vi "UNO_01.vi"() -> ()   [LabVIEW 2011]
uses:
  <vilib>/LabVIEW Interface for Arduino/Type Defs/Analog Pin.ctl
  <vilib>/LabVIEW Interface for Arduino/LabVIEW Interface for Arduino.lvlib
  <vilib>/Analysis/NI_AALBase.lvlib
panel:
  out "appended array 2":dbl[][](array[numeric])
  out "appended array":dbl[][](array[numeric])
  out "t":dbl[](array[numeric])
  out "path RLC":path
  out "MEASURE V [V]":dbl
  out "MEASURE I [A]":dbl
  out "MEASURE I [A]   2":dbl
  out "MEASURE V [V]  2":dbl
  out "MEASURE I [A]   8":dbl
  out "MEASURE V [V]  8":dbl
  out "MEASURE I [A]   7":dbl
  out "MEASURE V [V]  7":dbl
  out "MEASURE I [A]   6":dbl
  out "MEASURE V [V]  6":dbl
  out "MEASURE I [A]   5":dbl
  out "MEASURE V [V]  5":dbl
  out "MEASURE I [A]   4":dbl
  out "MEASURE V [V]  4":dbl
  out "MEASURE I [A]   3":dbl
  out "MEASURE V [V]  3":dbl
  out "MEASURE V [V]  16":dbl
  out "MEASURE I [A]   16":dbl
  out "MEASURE V [V]  15":dbl
  out "MEASURE I [A]   15":dbl
  out "MEASURE V [V]  14":dbl
  out "MEASURE I [A]   14":dbl
  out "MEASURE V [V]  13":dbl
  out "MEASURE I [A]   13":dbl
  out "MEASURE V [V]  12":dbl
  out "MEASURE I [A]   12":dbl
  out "MEASURE V [V]  11":dbl
  out "MEASURE I [A]   11":dbl
  out "MEASURE V [V]  10":dbl
  out "MEASURE I [A]   10":dbl
  out "MEASURE V [V]  9":dbl
  out "MEASURE I [A]   9":dbl
  out "RLC300 - digimess":string
  in  "dados":string
  in  "Tab Control":enum32{"Page 1", "Page 2"}(tab)
  out "Waveform Chart 2":dynamicdata(graph)
  out "Waveform Chart":dynamicdata(graph)
  in  "Analog Pin A":T1
  out "Voltage A":dbl(knob) scale=0.0..5.0
  in  "Analog Pin B":T1
  in  "Analog Pin C":T1
  out "Voltage B":dbl(knob) scale=0.0..5.0
  out "Voltage C":dbl(knob) scale=0.0..5.0
  out "Analog Port":dbl[](array[numeric])
  out "Resistencia":dbl
  out "Temperatura":dbl
  out "mean 2":dbl format="%.3p"
  in  "Refresh Button":bool
  out "Waveform Chart P 2":dbl[][](graph)
  out "C-50-N":bool
  out "C-50-L":bool
  out "Time":timestamp format="%<%X\n%x>T"
  out "Waveform Chart T":dynamicdata(graph)
  out "Waveform Chart P":dynamicdata(graph)
  out "Temperature (ºC)":dbl format="%#_4g"
  out "Pressure (bar)":dbl format="%#_4g"
  in  "New":bool
  in  "File name":string
  in  "Nota 01":string
  in  "Nota 2":string
  in  "Nota 3":string
  out "path":path
  in  "Sample name":string
  in  "Save Data":bool
  in  "Ajute P":dbl
  in  "Ajute T":dbl
  in  "Time (sec)":dbl
  in  "Stop":bool
  in  "New Button":bool
  in  "RLC":bool
  in  "Ligar RLC":bool
  in  "Close RLC 2":bool
  in  "read RLC":bool
  out "MEASURE A":dbl
  out "MEASURE B":dbl
  out "MEASURE B 2":dbl
  out "MEASURE A 2":dbl
  out "MEASURE B 8":dbl
  out "MEASURE A 8":dbl
  out "MEASURE B 7":dbl
  out "MEASURE A 7":dbl
  out "MEASURE B 6":dbl
  out "MEASURE A 6":dbl
  out "MEASURE B 5":dbl
  out "MEASURE A 5":dbl
  out "MEASURE B 4":dbl
  out "MEASURE A 4":dbl
  out "MEASURE B 3":dbl
  out "MEASURE A 3":dbl
  out "MEASURE B 9":dbl
  out "MEASURE A 9":dbl
  out "MEASURE B 10":dbl
  out "MEASURE A 10":dbl
  out "MEASURE B 11":dbl
  out "MEASURE A 11":dbl
  out "MEASURE B 12":dbl
  out "MEASURE A 12":dbl
  out "MEASURE B 13":dbl
  out "MEASURE A 13":dbl
  out "MEASURE B 14":dbl
  out "MEASURE A 14":dbl
  out "MEASURE B 15":dbl
  out "MEASURE A 15":dbl
  out "MEASURE B 16":dbl
  out "MEASURE A 16":dbl
  out "C-100-L":bool
  out "C-100-N":bool
  out "C-1K-L":bool
  out "C-1K-N":bool
  out "C-10K-L":bool
  out "C-10K-N":bool
  out "Z-50-L":bool
  out "Z-50-N":bool
  out "Z-100-L":bool
  out "Z-100-N":bool
  out "Z-1K-L":bool
  out "Z-1K-N":bool
  out "Z-10K-L":bool
  out "Z-10K-N":bool
  out "SET":dbl format="%#_3g"
  out "Waveform Chart P 3":dbl[][](graph)
  out "mean":dbl format="%.3p"
  out "mean 8":dbl format="%.3p"
  out "mean 7":dbl format="%.3p"
  out "mean 6":dbl format="%.3p"
  out "mean 5":dbl format="%.3p"
  out "mean 4":dbl format="%.3p"
  out "mean 3":dbl format="%.3p"
  out "mean 9":dbl format="%.3p"
  out "mean 10":dbl format="%.3p"
  out "mean 11":dbl format="%.3p"
  out "mean 12":dbl format="%.3p"
  out "mean 13":dbl format="%.3p"
  out "mean 14":dbl format="%.3p"
  out "mean 15":dbl format="%.3p"
  out "mean 16":dbl format="%.3p"
  # "C ( F )"
  # "R ( Ohm )"
  # "Z ( Ohm )"
  # "Phase ( deg)"
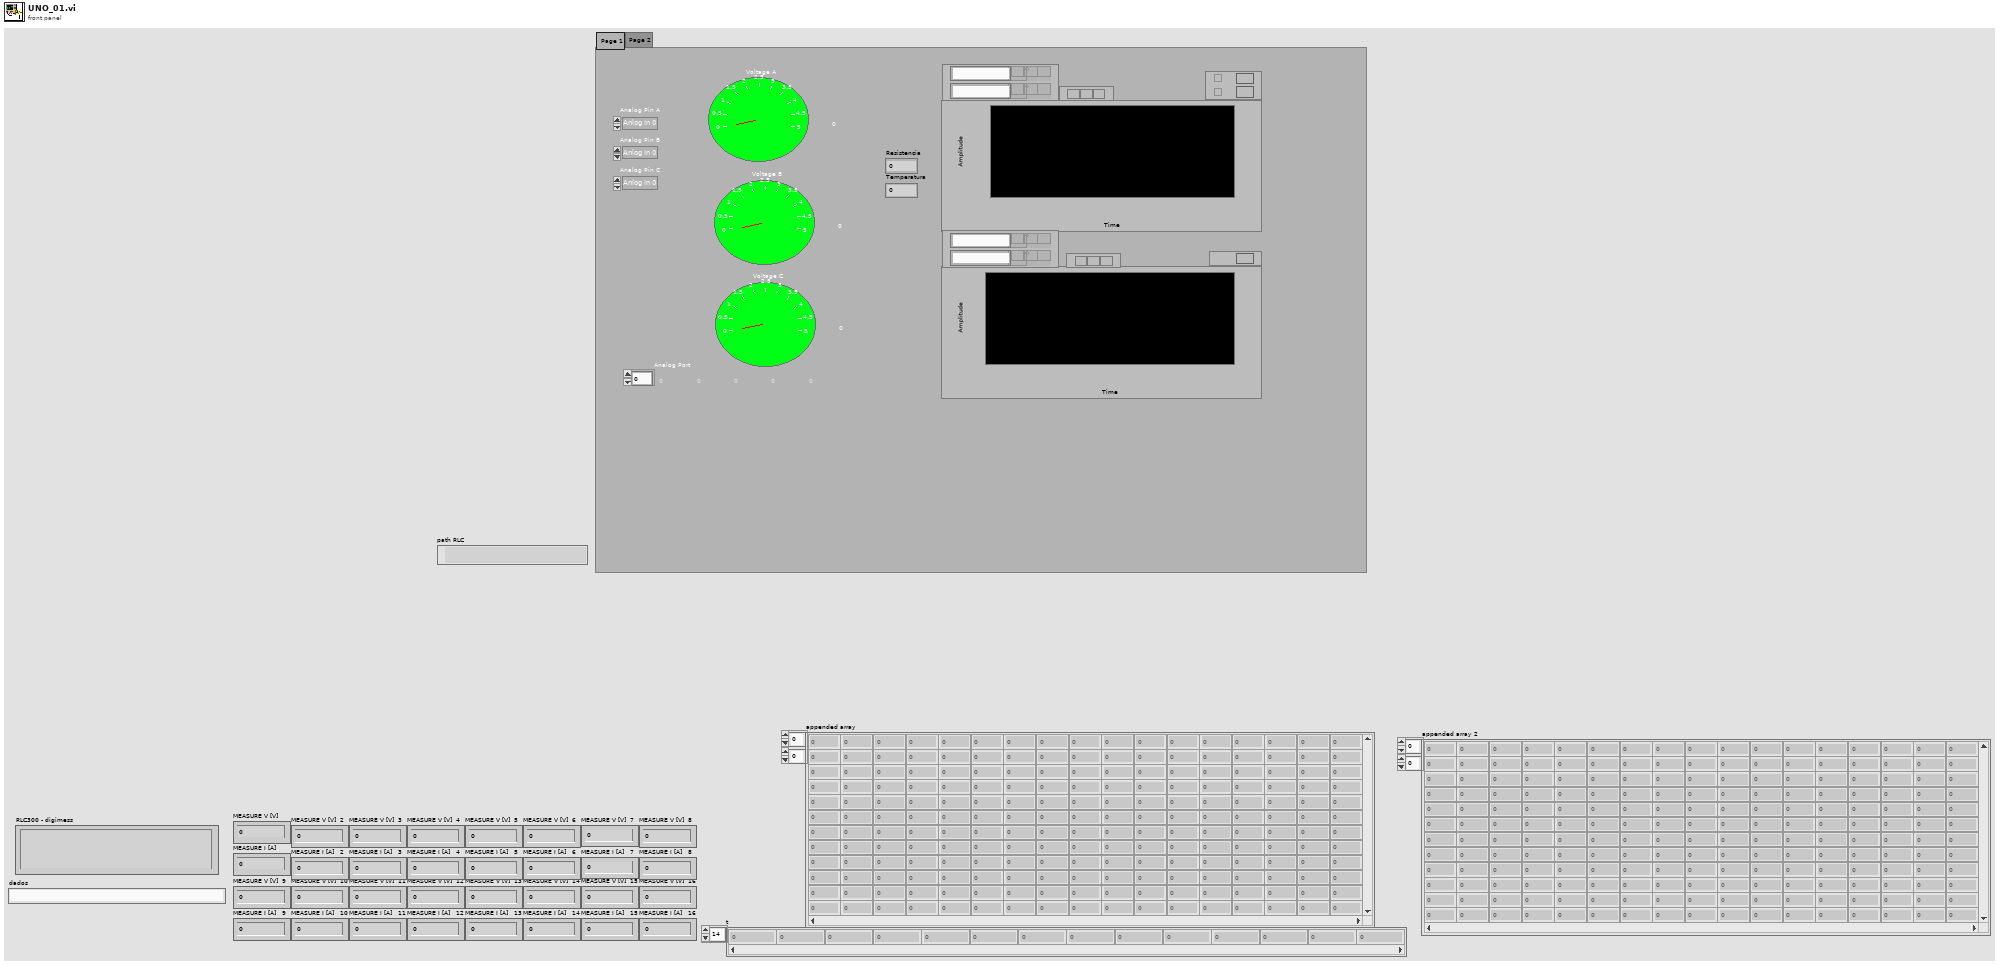
[diagram p1: front panel]
types:
  T1 = typedef "LabVIEW Interface for Arduino.lvlib/Analog Pin.ctl" = enum8{"Anlog In 0", "Anlog In 1", "Anlog In 2", "Anlog In 3", "Anlog In 4", "Anlog In 5"}
  T2 = typedef "LabVIEW Interface for Arduino.lvlib/Arduino Resource.ctl" = cluster{"VISA resource":refnum<visa-resource-name>, "Board Type":T3, "Connection Type":enum8{"USB / Serial"}, "Bytes Per Packet (15)":u8}
  T3 = typedef "LabVIEW Interface for Arduino.lvlib/Board Type.ctl" = enum16{"Uno", "Dimuelanove w/Atmega 328", "Mega 2560"}
  T4 = enum16{"open", "replace", "create", "open or create", "replace or create", "replace or create with confirmation"}
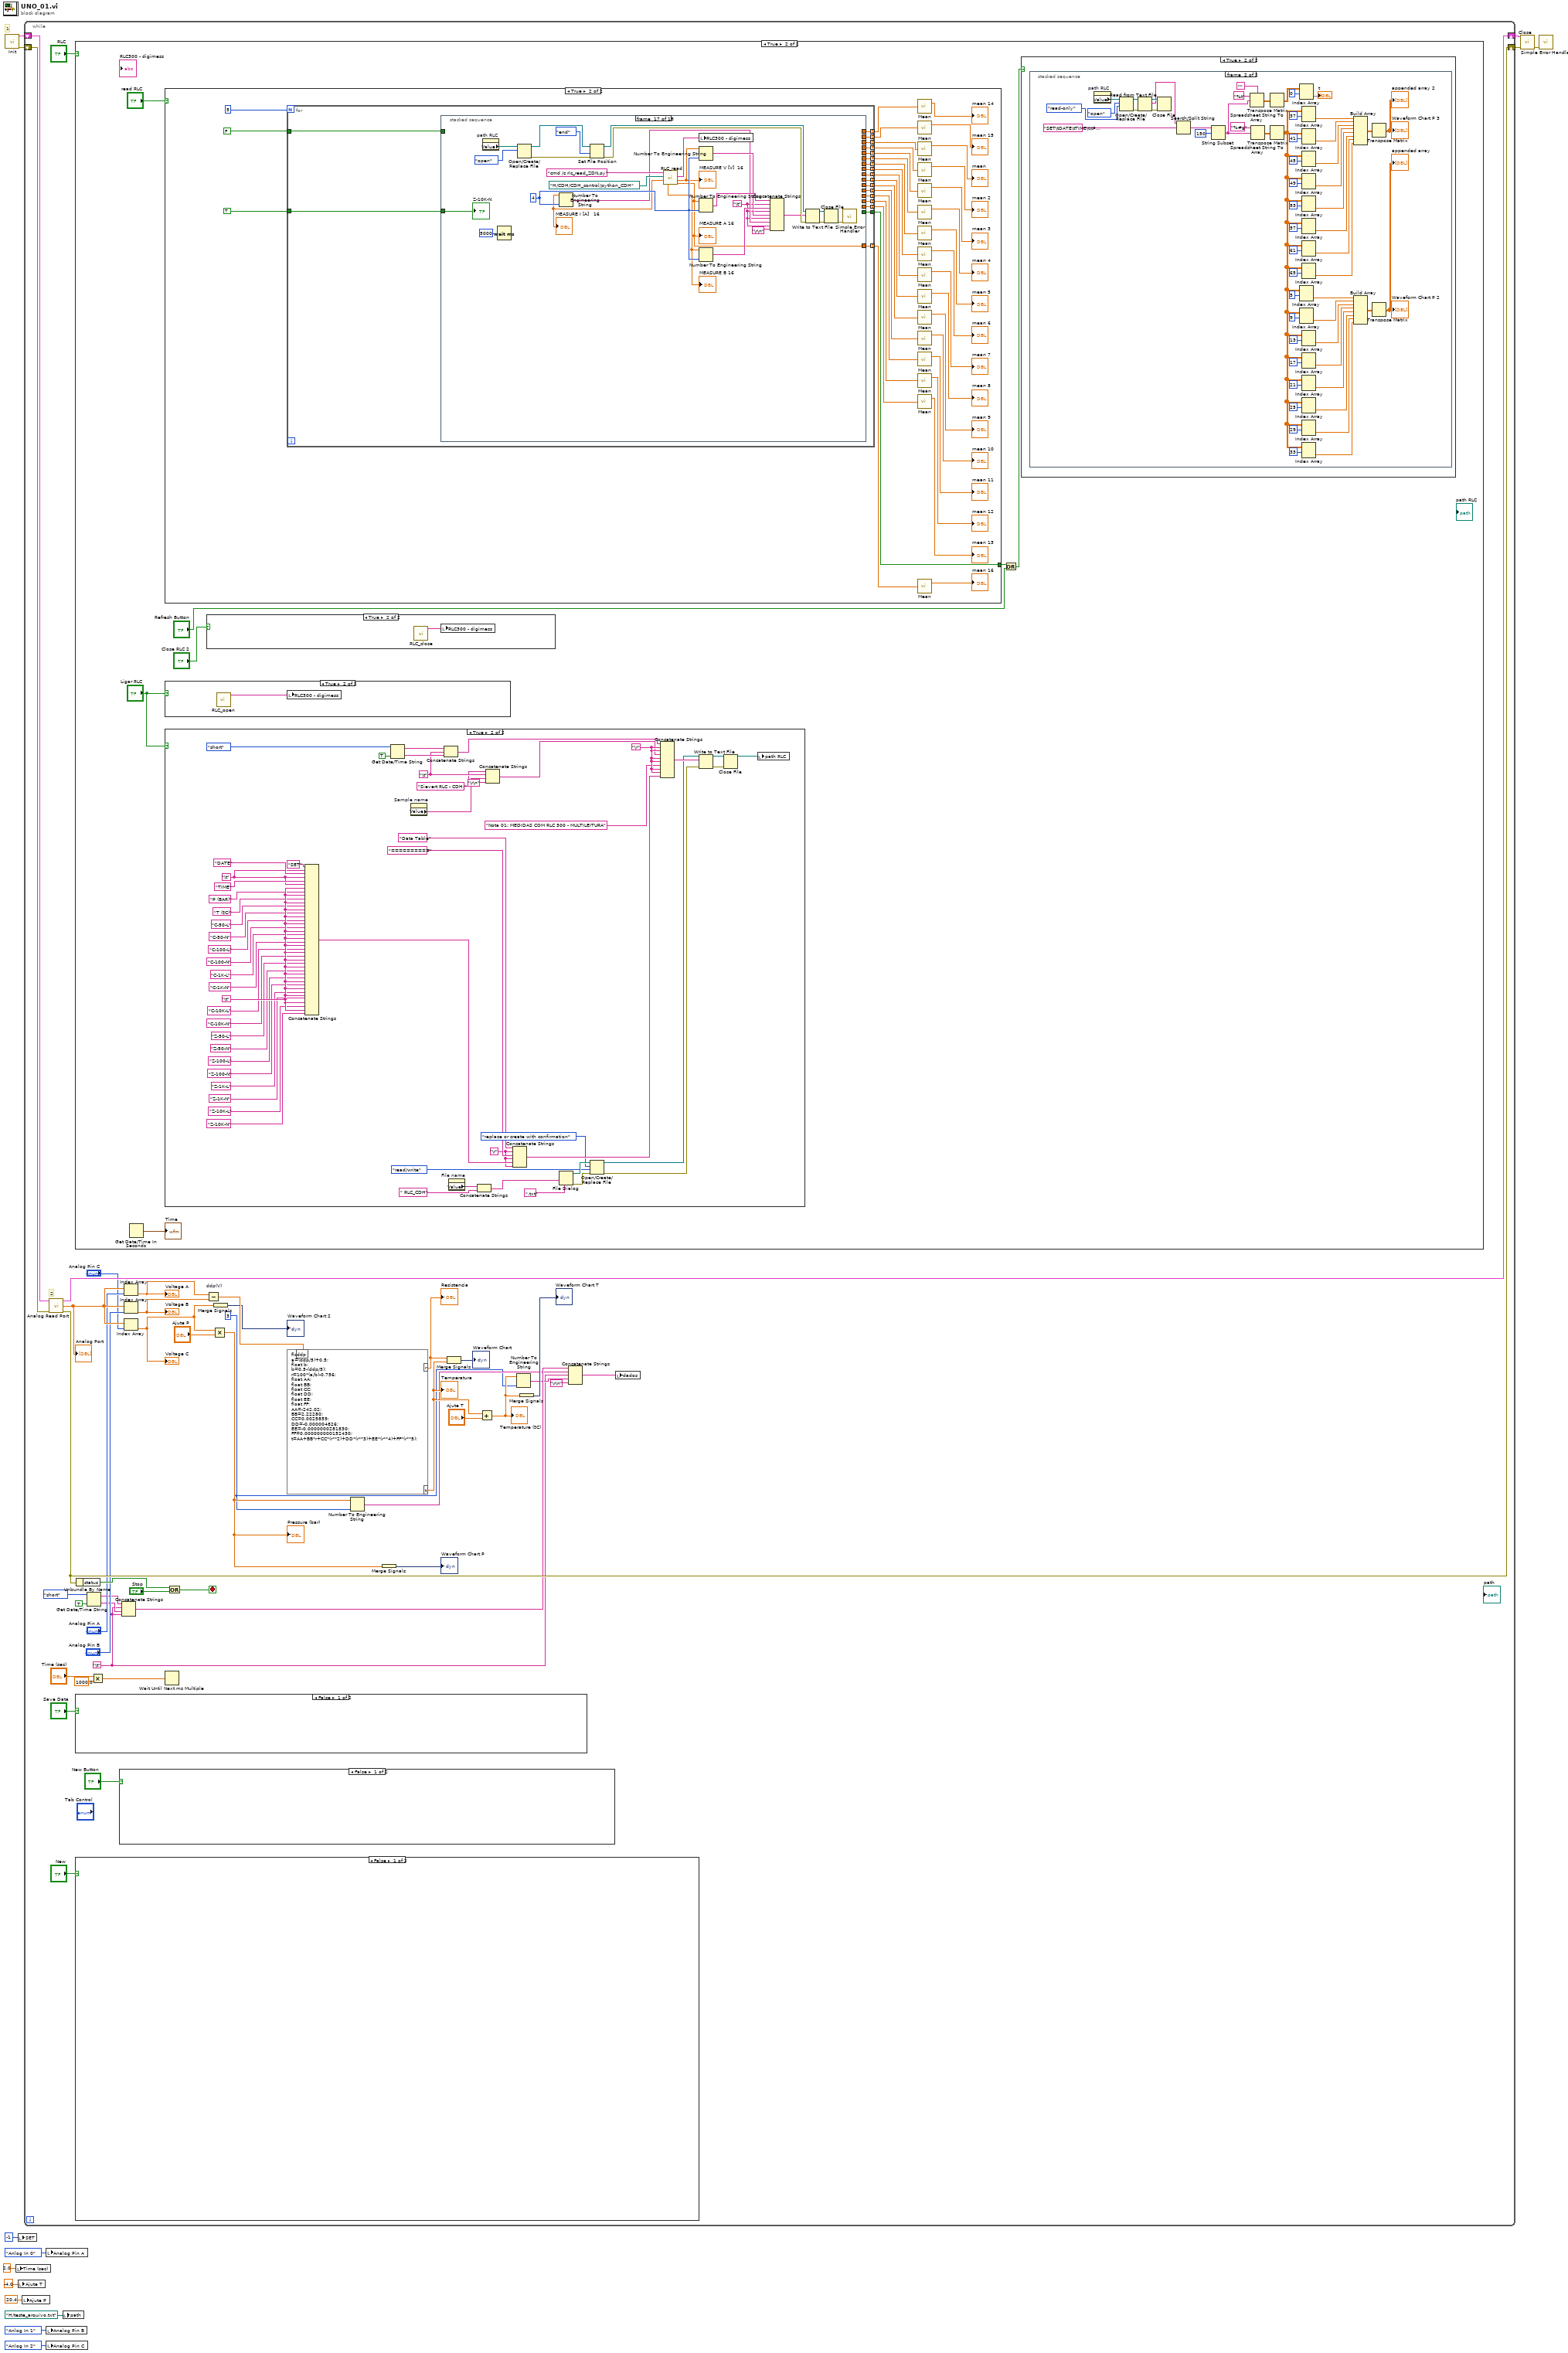
[diagram p0: block diagram]
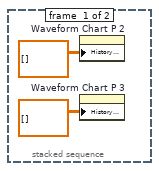
[diagram p4: hidden frame]
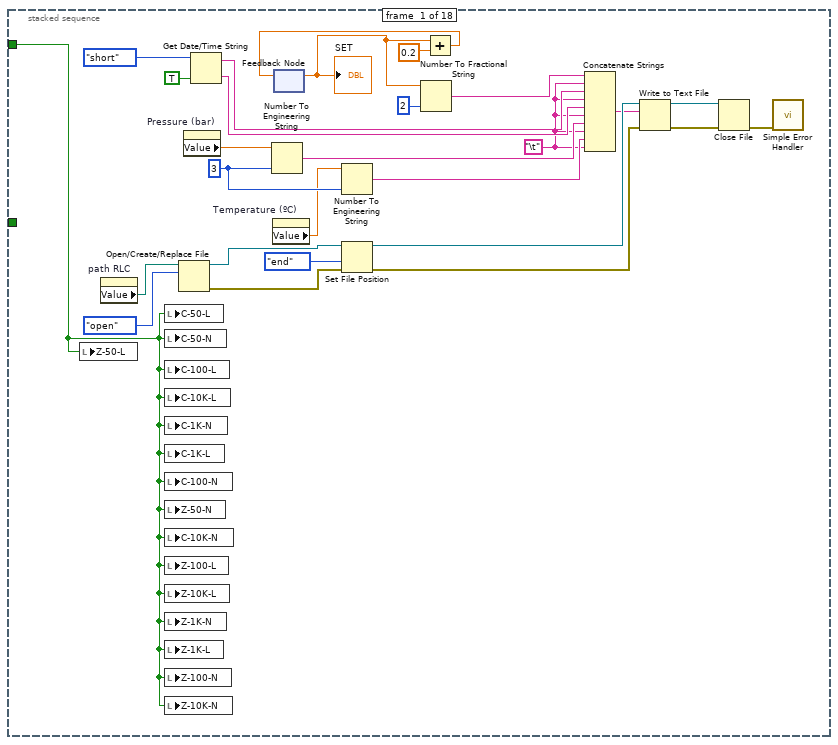
[diagram p7: hidden frame]
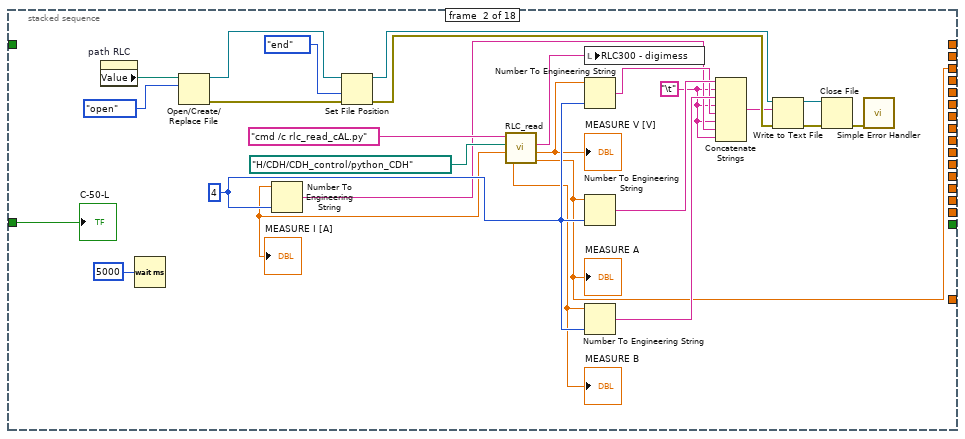
[diagram p8: hidden frame]
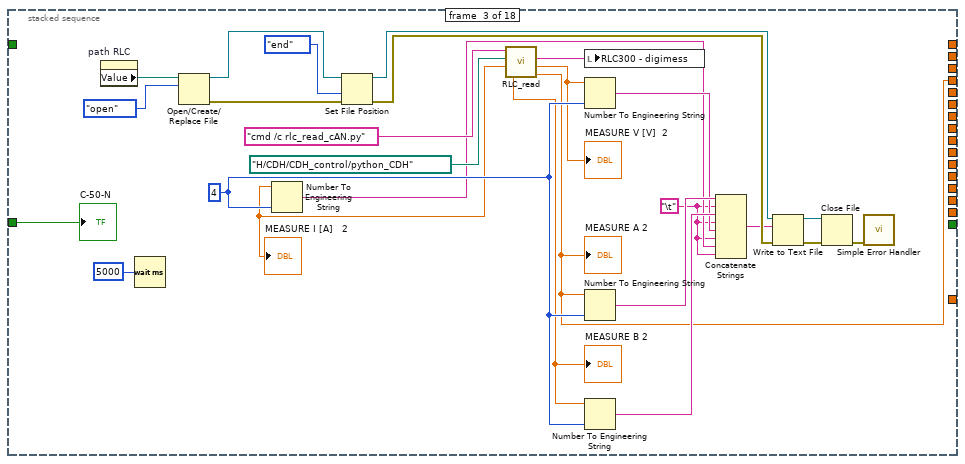
[diagram p9: hidden frame]
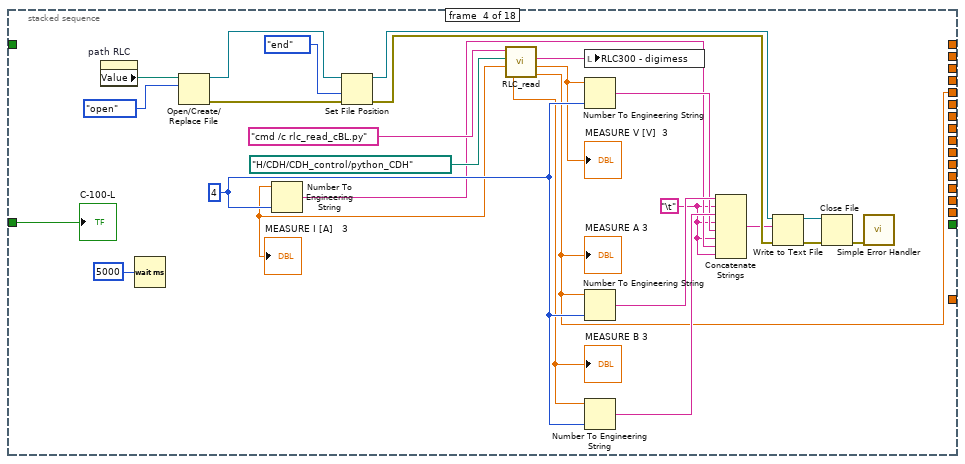
[diagram p10: hidden frame]
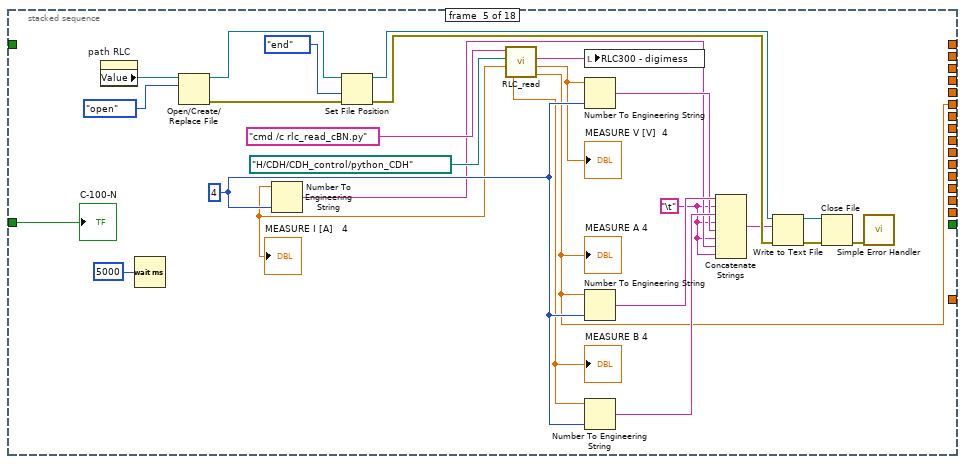
[diagram p11: hidden frame]
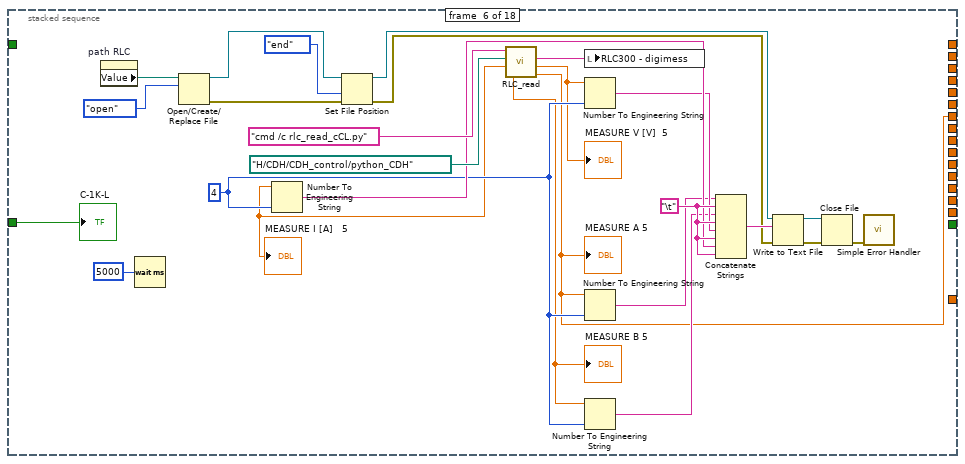
[diagram p12: hidden frame]
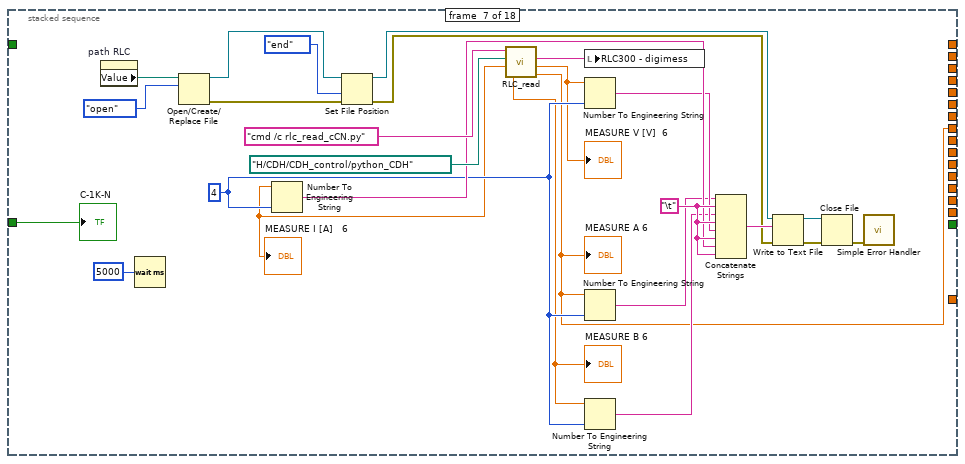
[diagram p13: hidden frame]
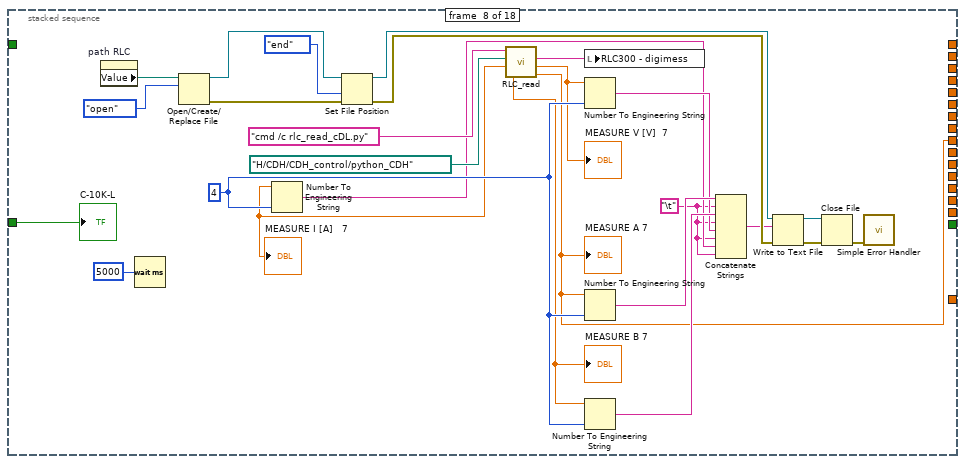
[diagram p14: hidden frame]
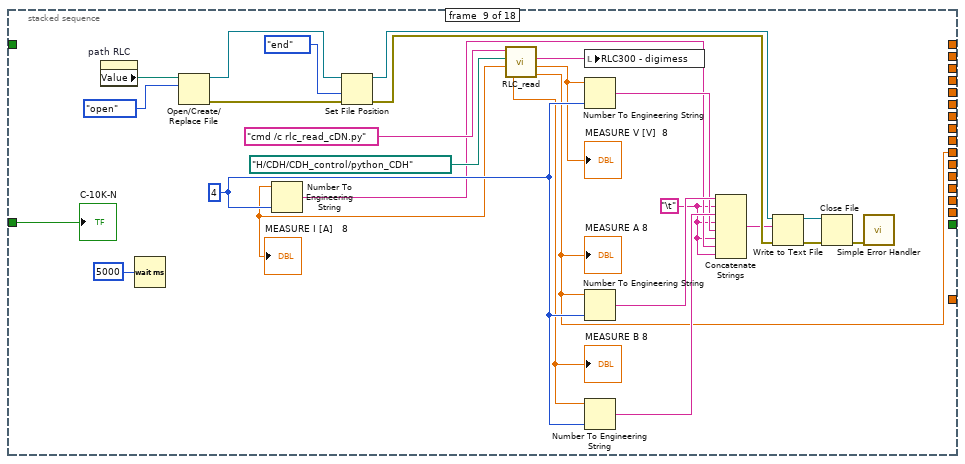
[diagram p15: hidden frame]
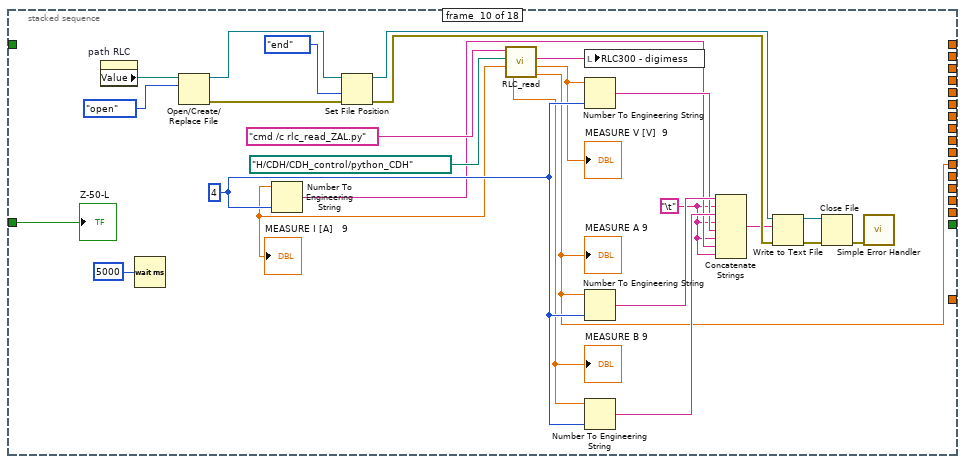
[diagram p16: hidden frame]
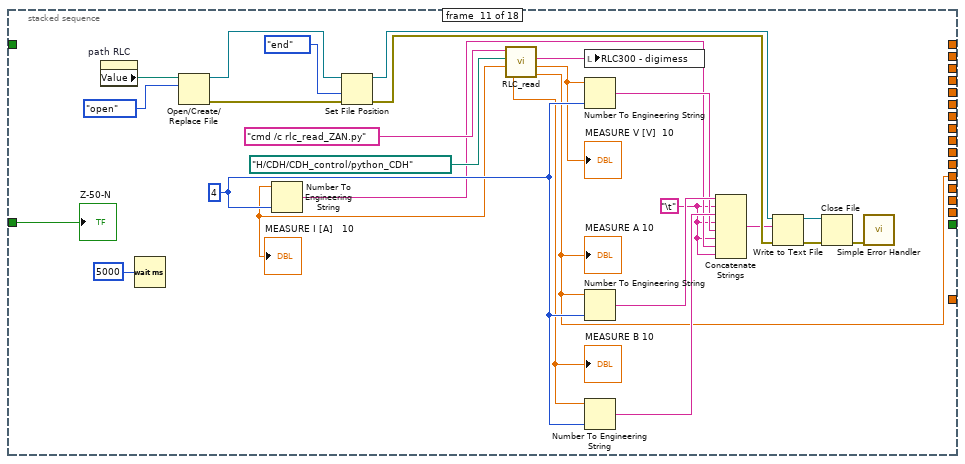
[diagram p17: hidden frame]
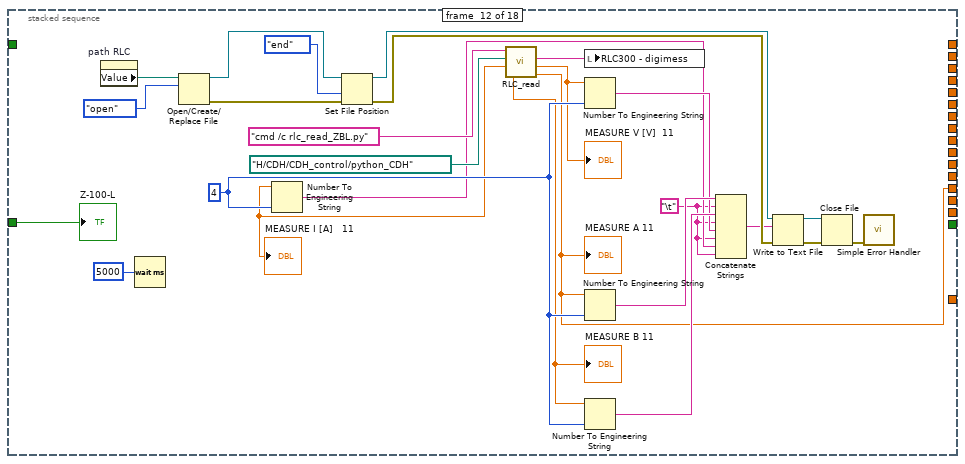
[diagram p18: hidden frame]
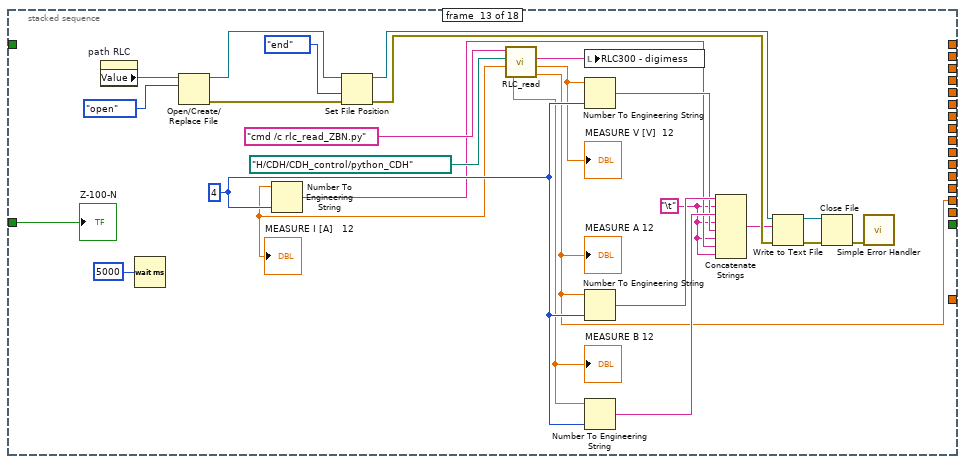
[diagram p19: hidden frame]
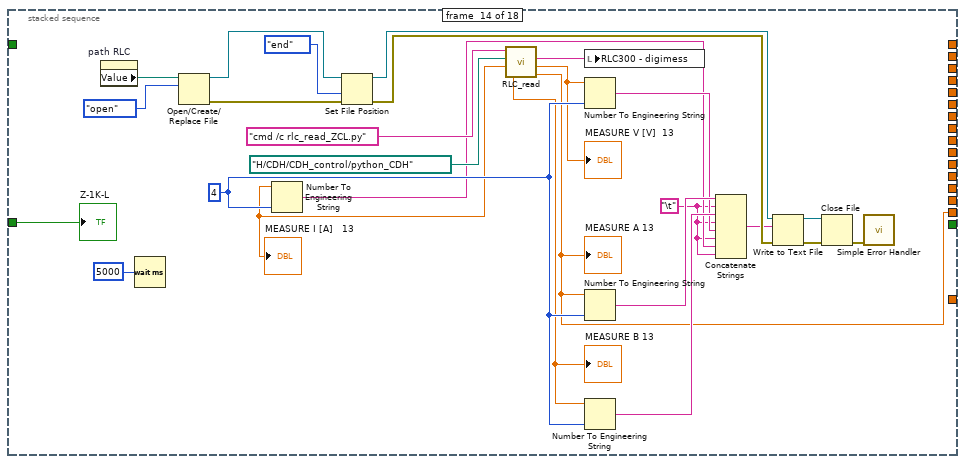
[diagram p20: hidden frame]
diagram:
  # "1"
  n1 = call <vilib>:"Init.vi"() -> ("Arduino Resource"=w13:T2, "error out"=w10:errorcluster)  [unwired: 18 in]
  n2 = local write "Time (sec)"(2.0 ("Time")) -> ()
  n3 = local write "SET"(-1 ("SET")) -> ()
  n4 = local write "Ajute T"(-4.0 ("Ajute T")) -> ()
  n5 = local write "Ajute P"(20.4 ("Ajute P")) -> ()
  n6 = while {
    shift-right: [w56] -> w12
    shift-left: w13 -> [w51]
    shift-right: [w55] -> w11
    shift-left: w10 -> [w50]
    stop <- w54 stop-if-true
    w16 = i16 3 ("width (-)")
    w17 = "\t"
    # "2"
    n7 = call <vilib>:"Analog Read Port.vi"("Arduino Resource"=w51, "error in"=w50) -> ("Arduino Resource"=w56:T2, "Analog Port"=w49:dbl[], "error out"=w55:errorcluster)  [unwired: 11 in]
    "Analog Port" <- w49
    n8 = case shown="True" "RLC" {
      frame False {
      }
      frame True {
        n9 = Get Date/Time In Seconds() -> (seconds since 1Jan1904=→"Time":timestamp)
        n10 = case shown="True" "read RLC" {
          tunnel: [_ w210] -> w57
          frame False {
          }
          frame True {
            n11 = for {
              N: 5 -> [_]
              tunnel: TRUE -> [w231]
              tunnel: FALSE -> [w230]
              tunnel: [w229] -> w210
              tunnel: [w228] -> w208 mode=indexing
              tunnel: [w227] -> w207 mode=indexing
              tunnel: [w226] -> w206 mode=indexing
              tunnel: [w225] -> w205 mode=indexing
              tunnel: [w224] -> w204 mode=indexing
              tunnel: [w223] -> w203 mode=indexing
              tunnel: [w222] -> w202 mode=indexing
              tunnel: [w221] -> w201 mode=indexing
              tunnel: [w220] -> w200 mode=indexing
              tunnel: [w219] -> w199 mode=indexing
              tunnel: [w218] -> w198 mode=indexing
              tunnel: [w217] -> w197 mode=indexing
              tunnel: [w216] -> w196 mode=indexing
              tunnel: [w215] -> w195 mode=indexing
              tunnel: [w214] -> w194 mode=indexing
              tunnel: [w213] -> w193 mode=indexing
              n12 = stacked-sequence {
                tunnel: w231 -> [_ w280 w306 w333 w358 w385 w410 w437 w463 w488 w514 w540 w566 w592 w618 w644 w671 _]
                tunnel: w230 -> [w258 _ _ _ _ _ _ _ _ _ _ _ _ _ _ _ _ w677]
                tunnel: [_ _ _ _ _ _ _ _ _ _ _ _ _ _ _ _ _ TRUE] -> w229
                tunnel: [_ w259 _ _ _ _ _ _ _ _ _ _ _ _ _ _ _ _] -> w228
                tunnel: [_ _ w285 _ _ _ _ _ _ _ _ _ _ _ _ _ _ _] -> w227
                tunnel: [_ _ _ w311 _ _ _ _ _ _ _ _ _ _ _ _ _ _] -> w226
                tunnel: [_ _ _ _ w337 _ _ _ _ _ _ _ _ _ _ _ _ _] -> w225
                tunnel: [_ _ _ _ _ w363 _ _ _ _ _ _ _ _ _ _ _ _] -> w224
                tunnel: [_ _ _ _ _ _ w389 _ _ _ _ _ _ _ _ _ _ _] -> w223
                tunnel: [_ _ _ _ _ _ _ w415 _ _ _ _ _ _ _ _ _ _] -> w222
                tunnel: [_ _ _ _ _ _ _ _ w441 _ _ _ _ _ _ _ _ _] -> w221
                tunnel: [_ _ _ _ _ _ _ _ _ w467 _ _ _ _ _ _ _ _] -> w220
                tunnel: [_ _ _ _ _ _ _ _ _ _ w493 _ _ _ _ _ _ _] -> w219
                tunnel: [_ _ _ _ _ _ _ _ _ _ _ w519 _ _ _ _ _ _] -> w218
                tunnel: [_ _ _ _ _ _ _ _ _ _ _ _ w545 _ _ _ _ _] -> w217
                tunnel: [_ _ _ _ _ _ _ _ _ _ _ _ _ w571 _ _ _ _] -> w216
                tunnel: [_ _ _ _ _ _ _ _ _ _ _ _ _ _ w597 _ _ _] -> w215
                tunnel: [_ _ _ _ _ _ _ _ _ _ _ _ _ _ _ w623 _ _] -> w214
                tunnel: [_ _ _ _ _ _ _ _ _ _ _ _ _ _ _ _ w649 _] -> w213
                frame #0 {
                  w237 = i16 3 ("width (-)")
                  w232 = "\t"
                  n13 = local write "Z-50-L"(w258) -> ()
                  n14 = property on="path RLC" class="Path"() -> ("Value"=w248:path)  [unwired: 2 in, 2 out]
                  n15 = local write "C-50-L"(w258) -> ()
                  n16 = local write "C-50-N"(w258) -> ()
                  n17 = local write "C-100-L"(w258) -> ()
                  n18 = local write "C-10K-L"(w258) -> ()
                  n19 = local write "C-1K-N"(w258) -> ()
                  n20 = local write "C-1K-L"(w258) -> ()
                  n21 = local write "C-100-N"(w258) -> ()
                  n22 = local write "Z-50-N"(w258) -> ()
                  n23 = local write "C-10K-N"(w258) -> ()
                  n24 = local write "Z-100-L"(w258) -> ()
                  n25 = local write "Z-10K-L"(w258) -> ()
                  n26 = local write "Z-1K-N"(w258) -> ()
                  n27 = local write "Z-1K-L"(w258) -> ()
                  n28 = local write "Z-100-N"(w258) -> ()
                  n29 = local write "Z-10K-N"(w258) -> ()
                  n30 = Open/Create/Replace File(file path (use dialog)=w248, operation (0:open)=T4."open") -> (refnum out=w252:refnum<file>, error out=w251:errorcluster)  [unwired: 2 in, 3 out]
                  n31 = property on="Pressure (bar)" class="DigNum (strict)"() -> ("Value"=w236:dbl)  [unwired: 2 in, 2 out]
                  n32 = Get Date/Time String(date format (0)=enum16{"short", "long", "abbreviated"}."short", want seconds? (F)=TRUE) -> (date string=w243:string, time string=w242:string)  [unwired: 1 in]
                  n33 = Number To Engineering String(2:w237, 4:w236) -> (0:w234:string)  [unwired: 2 in]
                  n34 = property on="Temperature (ºC)" class="DigNum (strict)"() -> ("Value"=w235:dbl)  [unwired: 2 in, 2 out]
                  n35 = feedback #1() -> (w241:dbl)  [unwired: 1 in]
                  "SET" <- w241
                  n36 = Number To Engineering String(2:w237, 4:w235) -> (0:w233:string)  [unwired: 2 in]
                  n37 = Set File Position(refnum=w252, from (0:start)=enum16{"start", "end", "current"}."end", error in=w251) -> (refnum out=w254:refnum<file>, error out=w255:errorcluster)  [unwired: 1 in]
                  n38 = Number To Fractional String(number=w241, precision (6)=i16 2) -> (F-format string=w240:string)  [unwired: 2 in]
                  n39 = Add(x=w241, y=0.2) -> (x+y=w247:dbl)
                  n40 = feedback-in #1(w247) -> ()
                  n41 = Concatenate Strings(w240, w232, w243, w232, w242, w232, w234, w232, w233, w232) -> (w239:string)
                  n42 = Write to Text File(file (use dialog)=w254, text=w239, error in=w255) -> (refnum out=w250:refnum<file>, error out=w249:errorcluster)  [unwired: 1 in, 1 out]
                  n43 = Close File(refnum=w250, error in=w249) -> (error out=w257:errorcluster)  [unwired: 1 out]
                  n44 = call <vilib>:"Simple Error Handler.vi"("error in (no error)"=w257) -> ()  [unwired: 1 in, 8 out]
                }
                frame #1 {
                  w260 = "\t"
                  w279 = i16 4 ("width (-)")
                  n45 = property on="path RLC" class="Path"() -> ("Value"=w265:path)  [unwired: 2 in, 2 out]
                  n46 = Wait (ms)(milliseconds to wait=u32 5000) -> ()  [unwired: 1 out]
                  n47 = Open/Create/Replace File(file path (use dialog)=w265, operation (0:open)=T4."open") -> (refnum out=w270:refnum<file>, error out=w269:errorcluster)  [unwired: 2 in, 3 out]
                  n48 = Set File Position(refnum=w270, from (0:start)=enum16{"start", "end", "current"}."end", error in=w269) -> (refnum out=w272:refnum<file>, error out=w273:errorcluster)  [unwired: 1 in]
                  n49 = call "RLC_read.vi"("Path"=path "H:/CDH/CDH_control/python_CDH", "String"="cmd /c rlc_read_cAL.py") -> ("MEASURE A"=w259:dbl, "MEASURE V [V]"=w277:dbl, "concatenated string"=w282:string, "MEASURE B"=w278:dbl, "MEASURE I [A]"=w276:dbl)  [unwired: 1 out]
                  "MEASURE A" <- w259
                  "MEASURE B" <- w278
                  "MEASURE V [V]" <- w277
                  "MEASURE I [A]" <- w276
                  n50 = Number To Engineering String(2:w279, 4:w276) -> (0:w261:string)  [unwired: 2 in]
                  n51 = local write "RLC300 - digimess"(w282) -> ()
                  n52 = Number To Engineering String(2:w279, 4:w277) -> (0:w262:string)  [unwired: 2 in]
                  n53 = Number To Engineering String(2:w279, 4:w259) -> (0:w264:string)  [unwired: 2 in]
                  n54 = Number To Engineering String(2:w279, 4:w278) -> (0:w263:string)  [unwired: 2 in]
                  n55 = Concatenate Strings(w264, w260, w263, w260, w262, w260, w261, w260) -> (w266:string)
                  n56 = Write to Text File(file (use dialog)=w272, text=w266, error in=w273) -> (refnum out=w268:refnum<file>, error out=w267:errorcluster)  [unwired: 1 in, 1 out]
                  n57 = Close File(refnum=w268, error in=w267) -> (error out=w275:errorcluster)  [unwired: 1 out]
                  n58 = call <vilib>:"Simple Error Handler.vi"("error in (no error)"=w275) -> ()  [unwired: 1 in, 8 out]
                  "C-50-L" <- w280
                }
                frame #2 {
                  w289 = "\t"
                  w305 = i16 4 ("width (-)")
                  n59 = property on="path RLC" class="Path"() -> ("Value"=w294:path)  [unwired: 2 in, 2 out]
                  n60 = Wait (ms)(milliseconds to wait=u32 5000) -> ()  [unwired: 1 out]
                  n61 = Open/Create/Replace File(file path (use dialog)=w294, operation (0:open)=T4."open") -> (refnum out=w299:refnum<file>, error out=w298:errorcluster)  [unwired: 2 in, 3 out]
                  n62 = Set File Position(refnum=w299, from (0:start)=enum16{"start", "end", "current"}."end", error in=w298) -> (refnum out=w301:refnum<file>, error out=w302:errorcluster)  [unwired: 1 in]
                  n63 = call "RLC_read.vi"("Path"=path "H:/CDH/CDH_control/python_CDH", "String"="cmd /c rlc_read_cAN.py") -> ("MEASURE A"=w285:dbl, "MEASURE V [V]"=w287:dbl, "concatenated string"=w309:string, "MEASURE B"=w288:dbl, "MEASURE I [A]"=w286:dbl)  [unwired: 1 out]
                  "MEASURE A 2" <- w285
                  "MEASURE B 2" <- w288
                  "MEASURE V [V]  2" <- w287
                  "MEASURE I [A]   2" <- w286
                  n64 = Number To Engineering String(2:w305, 4:w286) -> (0:w290:string)  [unwired: 2 in]
                  n65 = local write "RLC300 - digimess"(w309) -> ()
                  n66 = Number To Engineering String(2:w305, 4:w287) -> (0:w291:string)  [unwired: 2 in]
                  n67 = Number To Engineering String(2:w305, 4:w285) -> (0:w293:string)  [unwired: 2 in]
                  n68 = Number To Engineering String(2:w305, 4:w288) -> (0:w292:string)  [unwired: 2 in]
                  n69 = Concatenate Strings(w293, w289, w292, w289, w291, w289, w290, w289) -> (w295:string)
                  n70 = Write to Text File(file (use dialog)=w301, text=w295, error in=w302) -> (refnum out=w297:refnum<file>, error out=w296:errorcluster)  [unwired: 1 in, 1 out]
                  n71 = Close File(refnum=w297, error in=w296) -> (error out=w304:errorcluster)  [unwired: 1 out]
                  n72 = call <vilib>:"Simple Error Handler.vi"("error in (no error)"=w304) -> ()  [unwired: 1 in, 8 out]
                  "C-50-N" <- w306
                }
                frame #3 {
                  w315 = "\t"
                  w331 = i16 4 ("width (-)")
                  n73 = property on="path RLC" class="Path"() -> ("Value"=w320:path)  [unwired: 2 in, 2 out]
                  n74 = Wait (ms)(milliseconds to wait=u32 5000) -> ()  [unwired: 1 out]
                  n75 = Open/Create/Replace File(file path (use dialog)=w320, operation (0:open)=T4."open") -> (refnum out=w325:refnum<file>, error out=w324:errorcluster)  [unwired: 2 in, 3 out]
                  n76 = Set File Position(refnum=w325, from (0:start)=enum16{"start", "end", "current"}."end", error in=w324) -> (refnum out=w327:refnum<file>, error out=w328:errorcluster)  [unwired: 1 in]
                  n77 = call "RLC_read.vi"("Path"=path "H:/CDH/CDH_control/python_CDH", "String"="cmd /c rlc_read_cBL.py") -> ("MEASURE A"=w311:dbl, "MEASURE V [V]"=w313:dbl, "concatenated string"=w335:string, "MEASURE B"=w314:dbl, "MEASURE I [A]"=w312:dbl)  [unwired: 1 out]
                  "MEASURE A 3" <- w311
                  "MEASURE B 3" <- w314
                  "MEASURE V [V]  3" <- w313
                  "MEASURE I [A]   3" <- w312
                  n78 = Number To Engineering String(2:w331, 4:w312) -> (0:w316:string)  [unwired: 2 in]
                  n79 = local write "RLC300 - digimess"(w335) -> ()
                  n80 = Number To Engineering String(2:w331, 4:w313) -> (0:w317:string)  [unwired: 2 in]
                  n81 = Number To Engineering String(2:w331, 4:w311) -> (0:w319:string)  [unwired: 2 in]
                  n82 = Number To Engineering String(2:w331, 4:w314) -> (0:w318:string)  [unwired: 2 in]
                  n83 = Concatenate Strings(w319, w315, w318, w315, w317, w315, w316, w315) -> (w321:string)
                  n84 = Write to Text File(file (use dialog)=w327, text=w321, error in=w328) -> (refnum out=w323:refnum<file>, error out=w322:errorcluster)  [unwired: 1 in, 1 out]
                  n85 = Close File(refnum=w323, error in=w322) -> (error out=w330:errorcluster)  [unwired: 1 out]
                  n86 = call <vilib>:"Simple Error Handler.vi"("error in (no error)"=w330) -> ()  [unwired: 1 in, 8 out]
                  "C-100-L" <- w333
                }
                frame #4 {
                  w341 = "\t"
                  w357 = i16 4 ("width (-)")
                  n87 = property on="path RLC" class="Path"() -> ("Value"=w346:path)  [unwired: 2 in, 2 out]
                  n88 = Wait (ms)(milliseconds to wait=u32 5000) -> ()  [unwired: 1 out]
                  n89 = Open/Create/Replace File(file path (use dialog)=w346, operation (0:open)=T4."open") -> (refnum out=w351:refnum<file>, error out=w350:errorcluster)  [unwired: 2 in, 3 out]
                  n90 = Set File Position(refnum=w351, from (0:start)=enum16{"start", "end", "current"}."end", error in=w350) -> (refnum out=w353:refnum<file>, error out=w354:errorcluster)  [unwired: 1 in]
                  n91 = call "RLC_read.vi"("Path"=path "H:/CDH/CDH_control/python_CDH", "String"="cmd /c rlc_read_cBN.py") -> ("MEASURE A"=w337:dbl, "MEASURE V [V]"=w339:dbl, "concatenated string"=w361:string, "MEASURE B"=w340:dbl, "MEASURE I [A]"=w338:dbl)  [unwired: 1 out]
                  "MEASURE A 4" <- w337
                  "MEASURE B 4" <- w340
                  "MEASURE V [V]  4" <- w339
                  "MEASURE I [A]   4" <- w338
                  n92 = Number To Engineering String(2:w357, 4:w338) -> (0:w342:string)  [unwired: 2 in]
                  n93 = local write "RLC300 - digimess"(w361) -> ()
                  n94 = Number To Engineering String(2:w357, 4:w339) -> (0:w343:string)  [unwired: 2 in]
                  n95 = Number To Engineering String(2:w357, 4:w337) -> (0:w345:string)  [unwired: 2 in]
                  n96 = Number To Engineering String(2:w357, 4:w340) -> (0:w344:string)  [unwired: 2 in]
                  n97 = Concatenate Strings(w345, w341, w344, w341, w343, w341, w342, w341) -> (w347:string)
                  n98 = Write to Text File(file (use dialog)=w353, text=w347, error in=w354) -> (refnum out=w349:refnum<file>, error out=w348:errorcluster)  [unwired: 1 in, 1 out]
                  n99 = Close File(refnum=w349, error in=w348) -> (error out=w356:errorcluster)  [unwired: 1 out]
                  n100 = call <vilib>:"Simple Error Handler.vi"("error in (no error)"=w356) -> ()  [unwired: 1 in, 8 out]
                  "C-100-N" <- w358
                }
                frame #5 {
                  w383 = "\t"
                  w367 = i16 4 ("width (-)")
                  n101 = property on="path RLC" class="Path"() -> ("Value"=w378:path)  [unwired: 2 in, 2 out]
                  n102 = Wait (ms)(milliseconds to wait=u32 5000) -> ()  [unwired: 1 out]
                  n103 = Open/Create/Replace File(file path (use dialog)=w378, operation (0:open)=T4."open") -> (refnum out=w373:refnum<file>, error out=w374:errorcluster)  [unwired: 2 in, 3 out]
                  n104 = Set File Position(refnum=w373, from (0:start)=enum16{"start", "end", "current"}."end", error in=w374) -> (refnum out=w371:refnum<file>, error out=w370:errorcluster)  [unwired: 1 in]
                  n105 = call "RLC_read.vi"("Path"=path "H:/CDH/CDH_control/python_CDH", "String"="cmd /c rlc_read_cCL.py") -> ("MEASURE A"=w363:dbl, "MEASURE V [V]"=w365:dbl, "concatenated string"=w387:string, "MEASURE B"=w366:dbl, "MEASURE I [A]"=w364:dbl)  [unwired: 1 out]
                  "MEASURE A 5" <- w363
                  "MEASURE B 5" <- w366
                  "MEASURE V [V]  5" <- w365
                  "MEASURE I [A]   5" <- w364
                  n106 = Number To Engineering String(2:w367, 4:w364) -> (0:w382:string)  [unwired: 2 in]
                  n107 = local write "RLC300 - digimess"(w387) -> ()
                  n108 = Number To Engineering String(2:w367, 4:w365) -> (0:w381:string)  [unwired: 2 in]
                  n109 = Number To Engineering String(2:w367, 4:w363) -> (0:w379:string)  [unwired: 2 in]
                  n110 = Number To Engineering String(2:w367, 4:w366) -> (0:w380:string)  [unwired: 2 in]
                  n111 = Concatenate Strings(w379, w383, w380, w383, w381, w383, w382, w383) -> (w377:string)
                  n112 = Write to Text File(file (use dialog)=w371, text=w377, error in=w370) -> (refnum out=w375:refnum<file>, error out=w376:errorcluster)  [unwired: 1 in, 1 out]
                  n113 = Close File(refnum=w375, error in=w376) -> (error out=w368:errorcluster)  [unwired: 1 out]
                  n114 = call <vilib>:"Simple Error Handler.vi"("error in (no error)"=w368) -> ()  [unwired: 1 in, 8 out]
                  "C-1K-L" <- w385
                }
                frame #6 {
                  w409 = "\t"
                  w393 = i16 4 ("width (-)")
                  n115 = property on="path RLC" class="Path"() -> ("Value"=w404:path)  [unwired: 2 in, 2 out]
                  n116 = Wait (ms)(milliseconds to wait=u32 5000) -> ()  [unwired: 1 out]
                  n117 = Open/Create/Replace File(file path (use dialog)=w404, operation (0:open)=T4."open") -> (refnum out=w399:refnum<file>, error out=w400:errorcluster)  [unwired: 2 in, 3 out]
                  n118 = Set File Position(refnum=w399, from (0:start)=enum16{"start", "end", "current"}."end", error in=w400) -> (refnum out=w397:refnum<file>, error out=w396:errorcluster)  [unwired: 1 in]
                  n119 = call "RLC_read.vi"("Path"=path "H:/CDH/CDH_control/python_CDH", "String"="cmd /c rlc_read_cCN.py") -> ("MEASURE A"=w389:dbl, "MEASURE V [V]"=w391:dbl, "concatenated string"=w413:string, "MEASURE B"=w392:dbl, "MEASURE I [A]"=w390:dbl)  [unwired: 1 out]
                  "MEASURE A 6" <- w389
                  "MEASURE B 6" <- w392
                  "MEASURE V [V]  6" <- w391
                  "MEASURE I [A]   6" <- w390
                  n120 = Number To Engineering String(2:w393, 4:w390) -> (0:w408:string)  [unwired: 2 in]
                  n121 = local write "RLC300 - digimess"(w413) -> ()
                  n122 = Number To Engineering String(2:w393, 4:w391) -> (0:w407:string)  [unwired: 2 in]
                  n123 = Number To Engineering String(2:w393, 4:w389) -> (0:w405:string)  [unwired: 2 in]
                  n124 = Number To Engineering String(2:w393, 4:w392) -> (0:w406:string)  [unwired: 2 in]
                  n125 = Concatenate Strings(w405, w409, w406, w409, w407, w409, w408, w409) -> (w403:string)
                  n126 = Write to Text File(file (use dialog)=w397, text=w403, error in=w396) -> (refnum out=w401:refnum<file>, error out=w402:errorcluster)  [unwired: 1 in, 1 out]
                  n127 = Close File(refnum=w401, error in=w402) -> (error out=w394:errorcluster)  [unwired: 1 out]
                  n128 = call <vilib>:"Simple Error Handler.vi"("error in (no error)"=w394) -> ()  [unwired: 1 in, 8 out]
                  "C-1K-N" <- w410
                }
                frame #7 {
                  w419 = "\t"
                  w435 = i16 4 ("width (-)")
                  n129 = property on="path RLC" class="Path"() -> ("Value"=w424:path)  [unwired: 2 in, 2 out]
                  n130 = Wait (ms)(milliseconds to wait=u32 5000) -> ()  [unwired: 1 out]
                  n131 = Open/Create/Replace File(file path (use dialog)=w424, operation (0:open)=T4."open") -> (refnum out=w429:refnum<file>, error out=w428:errorcluster)  [unwired: 2 in, 3 out]
                  n132 = Set File Position(refnum=w429, from (0:start)=enum16{"start", "end", "current"}."end", error in=w428) -> (refnum out=w431:refnum<file>, error out=w432:errorcluster)  [unwired: 1 in]
                  n133 = call "RLC_read.vi"("Path"=path "H:/CDH/CDH_control/python_CDH", "String"="cmd /c rlc_read_cDL.py") -> ("MEASURE A"=w415:dbl, "MEASURE V [V]"=w417:dbl, "concatenated string"=w439:string, "MEASURE B"=w418:dbl, "MEASURE I [A]"=w416:dbl)  [unwired: 1 out]
                  "MEASURE A 7" <- w415
                  "MEASURE B 7" <- w418
                  "MEASURE V [V]  7" <- w417
                  "MEASURE I [A]   7" <- w416
                  n134 = Number To Engineering String(2:w435, 4:w416) -> (0:w420:string)  [unwired: 2 in]
                  n135 = local write "RLC300 - digimess"(w439) -> ()
                  n136 = Number To Engineering String(2:w435, 4:w417) -> (0:w421:string)  [unwired: 2 in]
                  n137 = Number To Engineering String(2:w435, 4:w415) -> (0:w423:string)  [unwired: 2 in]
                  n138 = Number To Engineering String(2:w435, 4:w418) -> (0:w422:string)  [unwired: 2 in]
                  n139 = Concatenate Strings(w423, w419, w422, w419, w421, w419, w420, w419) -> (w425:string)
                  n140 = Write to Text File(file (use dialog)=w431, text=w425, error in=w432) -> (refnum out=w427:refnum<file>, error out=w426:errorcluster)  [unwired: 1 in, 1 out]
                  n141 = Close File(refnum=w427, error in=w426) -> (error out=w434:errorcluster)  [unwired: 1 out]
                  n142 = call <vilib>:"Simple Error Handler.vi"("error in (no error)"=w434) -> ()  [unwired: 1 in, 8 out]
                  "C-10K-L" <- w437
                }
                frame #8 {
                  w445 = "\t"
                  w461 = i16 4 ("width (-)")
                  n143 = property on="path RLC" class="Path"() -> ("Value"=w450:path)  [unwired: 2 in, 2 out]
                  n144 = Wait (ms)(milliseconds to wait=u32 5000) -> ()  [unwired: 1 out]
                  n145 = Open/Create/Replace File(file path (use dialog)=w450, operation (0:open)=T4."open") -> (refnum out=w455:refnum<file>, error out=w454:errorcluster)  [unwired: 2 in, 3 out]
                  n146 = Set File Position(refnum=w455, from (0:start)=enum16{"start", "end", "current"}."end", error in=w454) -> (refnum out=w457:refnum<file>, error out=w458:errorcluster)  [unwired: 1 in]
                  n147 = call "RLC_read.vi"("Path"=path "H:/CDH/CDH_control/python_CDH", "String"="cmd /c rlc_read_cDN.py") -> ("MEASURE A"=w441:dbl, "MEASURE V [V]"=w443:dbl, "concatenated string"=w465:string, "MEASURE B"=w444:dbl, "MEASURE I [A]"=w442:dbl)  [unwired: 1 out]
                  "MEASURE A 8" <- w441
                  "MEASURE B 8" <- w444
                  "MEASURE V [V]  8" <- w443
                  "MEASURE I [A]   8" <- w442
                  n148 = Number To Engineering String(2:w461, 4:w442) -> (0:w446:string)  [unwired: 2 in]
                  n149 = local write "RLC300 - digimess"(w465) -> ()
                  n150 = Number To Engineering String(2:w461, 4:w443) -> (0:w447:string)  [unwired: 2 in]
                  n151 = Number To Engineering String(2:w461, 4:w441) -> (0:w449:string)  [unwired: 2 in]
                  n152 = Number To Engineering String(2:w461, 4:w444) -> (0:w448:string)  [unwired: 2 in]
                  n153 = Concatenate Strings(w449, w445, w448, w445, w447, w445, w446, w445) -> (w451:string)
                  n154 = Write to Text File(file (use dialog)=w457, text=w451, error in=w458) -> (refnum out=w453:refnum<file>, error out=w452:errorcluster)  [unwired: 1 in, 1 out]
                  n155 = Close File(refnum=w453, error in=w452) -> (error out=w460:errorcluster)  [unwired: 1 out]
                  n156 = call <vilib>:"Simple Error Handler.vi"("error in (no error)"=w460) -> ()  [unwired: 1 in, 8 out]
                  "C-10K-N" <- w463
                }
                frame #9 {
                  w471 = "\t"
                  w487 = i16 4 ("width (-)")
                  n157 = property on="path RLC" class="Path"() -> ("Value"=w476:path)  [unwired: 2 in, 2 out]
                  n158 = Wait (ms)(milliseconds to wait=u32 5000) -> ()  [unwired: 1 out]
                  n159 = Open/Create/Replace File(file path (use dialog)=w476, operation (0:open)=T4."open") -> (refnum out=w481:refnum<file>, error out=w480:errorcluster)  [unwired: 2 in, 3 out]
                  n160 = Set File Position(refnum=w481, from (0:start)=enum16{"start", "end", "current"}."end", error in=w480) -> (refnum out=w483:refnum<file>, error out=w484:errorcluster)  [unwired: 1 in]
                  n161 = call "RLC_read.vi"("Path"=path "H:/CDH/CDH_control/python_CDH", "String"="cmd /c rlc_read_ZAL.py") -> ("MEASURE A"=w467:dbl, "MEASURE V [V]"=w469:dbl, "concatenated string"=w490:string, "MEASURE B"=w470:dbl, "MEASURE I [A]"=w468:dbl)  [unwired: 1 out]
                  "MEASURE A 9" <- w467
                  "MEASURE B 9" <- w470
                  "MEASURE V [V]  9" <- w469
                  "MEASURE I [A]   9" <- w468
                  n162 = Number To Engineering String(2:w487, 4:w468) -> (0:w472:string)  [unwired: 2 in]
                  n163 = local write "RLC300 - digimess"(w490) -> ()
                  n164 = Number To Engineering String(2:w487, 4:w469) -> (0:w473:string)  [unwired: 2 in]
                  n165 = Number To Engineering String(2:w487, 4:w467) -> (0:w475:string)  [unwired: 2 in]
                  n166 = Number To Engineering String(2:w487, 4:w470) -> (0:w474:string)  [unwired: 2 in]
                  n167 = Concatenate Strings(w475, w471, w474, w471, w473, w471, w472, w471) -> (w477:string)
                  n168 = Write to Text File(file (use dialog)=w483, text=w477, error in=w484) -> (refnum out=w479:refnum<file>, error out=w478:errorcluster)  [unwired: 1 in, 1 out]
                  n169 = Close File(refnum=w479, error in=w478) -> (error out=w486:errorcluster)  [unwired: 1 out]
                  n170 = call <vilib>:"Simple Error Handler.vi"("error in (no error)"=w486) -> ()  [unwired: 1 in, 8 out]
                  "Z-50-L" <- w488
                }
                frame #10 {
                  w497 = "\t"
                  w513 = i16 4 ("width (-)")
                  n171 = property on="path RLC" class="Path"() -> ("Value"=w502:path)  [unwired: 2 in, 2 out]
                  n172 = Wait (ms)(milliseconds to wait=u32 5000) -> ()  [unwired: 1 out]
                  n173 = Open/Create/Replace File(file path (use dialog)=w502, operation (0:open)=T4."open") -> (refnum out=w507:refnum<file>, error out=w506:errorcluster)  [unwired: 2 in, 3 out]
                  n174 = Set File Position(refnum=w507, from (0:start)=enum16{"start", "end", "current"}."end", error in=w506) -> (refnum out=w509:refnum<file>, error out=w510:errorcluster)  [unwired: 1 in]
                  n175 = call "RLC_read.vi"("Path"=path "H:/CDH/CDH_control/python_CDH", "String"="cmd /c rlc_read_ZAN.py") -> ("MEASURE A"=w493:dbl, "MEASURE V [V]"=w495:dbl, "concatenated string"=w516:string, "MEASURE B"=w496:dbl, "MEASURE I [A]"=w494:dbl)  [unwired: 1 out]
                  "MEASURE A 10" <- w493
                  "MEASURE B 10" <- w496
                  "MEASURE V [V]  10" <- w495
                  "MEASURE I [A]   10" <- w494
                  n176 = Number To Engineering String(2:w513, 4:w494) -> (0:w498:string)  [unwired: 2 in]
                  n177 = local write "RLC300 - digimess"(w516) -> ()
                  n178 = Number To Engineering String(2:w513, 4:w495) -> (0:w499:string)  [unwired: 2 in]
                  n179 = Number To Engineering String(2:w513, 4:w493) -> (0:w501:string)  [unwired: 2 in]
                  n180 = Number To Engineering String(2:w513, 4:w496) -> (0:w500:string)  [unwired: 2 in]
                  n181 = Concatenate Strings(w501, w497, w500, w497, w499, w497, w498, w497) -> (w503:string)
                  n182 = Write to Text File(file (use dialog)=w509, text=w503, error in=w510) -> (refnum out=w505:refnum<file>, error out=w504:errorcluster)  [unwired: 1 in, 1 out]
                  n183 = Close File(refnum=w505, error in=w504) -> (error out=w512:errorcluster)  [unwired: 1 out]
                  n184 = call <vilib>:"Simple Error Handler.vi"("error in (no error)"=w512) -> ()  [unwired: 1 in, 8 out]
                  "Z-50-N" <- w514
                }
                frame #11 {
                  w523 = "\t"
                  w539 = i16 4 ("width (-)")
                  n185 = property on="path RLC" class="Path"() -> ("Value"=w528:path)  [unwired: 2 in, 2 out]
                  n186 = Wait (ms)(milliseconds to wait=u32 5000) -> ()  [unwired: 1 out]
                  n187 = Open/Create/Replace File(file path (use dialog)=w528, operation (0:open)=T4."open") -> (refnum out=w533:refnum<file>, error out=w532:errorcluster)  [unwired: 2 in, 3 out]
                  n188 = Set File Position(refnum=w533, from (0:start)=enum16{"start", "end", "current"}."end", error in=w532) -> (refnum out=w535:refnum<file>, error out=w536:errorcluster)  [unwired: 1 in]
                  n189 = call "RLC_read.vi"("Path"=path "H:/CDH/CDH_control/python_CDH", "String"="cmd /c rlc_read_ZBL.py") -> ("MEASURE A"=w519:dbl, "MEASURE V [V]"=w521:dbl, "concatenated string"=w542:string, "MEASURE B"=w522:dbl, "MEASURE I [A]"=w520:dbl)  [unwired: 1 out]
                  "MEASURE A 11" <- w519
                  "MEASURE B 11" <- w522
                  "MEASURE V [V]  11" <- w521
                  "MEASURE I [A]   11" <- w520
                  n190 = Number To Engineering String(2:w539, 4:w520) -> (0:w524:string)  [unwired: 2 in]
                  n191 = local write "RLC300 - digimess"(w542) -> ()
                  n192 = Number To Engineering String(2:w539, 4:w521) -> (0:w525:string)  [unwired: 2 in]
                  n193 = Number To Engineering String(2:w539, 4:w519) -> (0:w527:string)  [unwired: 2 in]
                  n194 = Number To Engineering String(2:w539, 4:w522) -> (0:w526:string)  [unwired: 2 in]
                  n195 = Concatenate Strings(w527, w523, w526, w523, w525, w523, w524, w523) -> (w529:string)
                  n196 = Write to Text File(file (use dialog)=w535, text=w529, error in=w536) -> (refnum out=w531:refnum<file>, error out=w530:errorcluster)  [unwired: 1 in, 1 out]
                  n197 = Close File(refnum=w531, error in=w530) -> (error out=w538:errorcluster)  [unwired: 1 out]
                  n198 = call <vilib>:"Simple Error Handler.vi"("error in (no error)"=w538) -> ()  [unwired: 1 in, 8 out]
                  "Z-100-L" <- w540
                }
                frame #12 {
                  w549 = "\t"
                  w565 = i16 4 ("width (-)")
                  n199 = property on="path RLC" class="Path"() -> ("Value"=w554:path)  [unwired: 2 in, 2 out]
                  n200 = Wait (ms)(milliseconds to wait=u32 5000) -> ()  [unwired: 1 out]
                  n201 = Open/Create/Replace File(file path (use dialog)=w554, operation (0:open)=T4."open") -> (refnum out=w559:refnum<file>, error out=w558:errorcluster)  [unwired: 2 in, 3 out]
                  n202 = Set File Position(refnum=w559, from (0:start)=enum16{"start", "end", "current"}."end", error in=w558) -> (refnum out=w561:refnum<file>, error out=w562:errorcluster)  [unwired: 1 in]
                  n203 = call "RLC_read.vi"("Path"=path "H:/CDH/CDH_control/python_CDH", "String"="cmd /c rlc_read_ZBN.py") -> ("MEASURE A"=w545:dbl, "MEASURE V [V]"=w547:dbl, "concatenated string"=w568:string, "MEASURE B"=w548:dbl, "MEASURE I [A]"=w546:dbl)  [unwired: 1 out]
                  "MEASURE A 12" <- w545
                  "MEASURE B 12" <- w548
                  "MEASURE V [V]  12" <- w547
                  "MEASURE I [A]   12" <- w546
                  n204 = Number To Engineering String(2:w565, 4:w546) -> (0:w550:string)  [unwired: 2 in]
                  n205 = local write "RLC300 - digimess"(w568) -> ()
                  n206 = Number To Engineering String(2:w565, 4:w547) -> (0:w551:string)  [unwired: 2 in]
                  n207 = Number To Engineering String(2:w565, 4:w545) -> (0:w553:string)  [unwired: 2 in]
                  n208 = Number To Engineering String(2:w565, 4:w548) -> (0:w552:string)  [unwired: 2 in]
                  n209 = Concatenate Strings(w553, w549, w552, w549, w551, w549, w550, w549) -> (w555:string)
                  n210 = Write to Text File(file (use dialog)=w561, text=w555, error in=w562) -> (refnum out=w557:refnum<file>, error out=w556:errorcluster)  [unwired: 1 in, 1 out]
                  n211 = Close File(refnum=w557, error in=w556) -> (error out=w564:errorcluster)  [unwired: 1 out]
                  n212 = call <vilib>:"Simple Error Handler.vi"("error in (no error)"=w564) -> ()  [unwired: 1 in, 8 out]
                  "Z-100-N" <- w566
                }
                frame #13 {
                  w575 = "\t"
                  w591 = i16 4 ("width (-)")
                  n213 = property on="path RLC" class="Path"() -> ("Value"=w580:path)  [unwired: 2 in, 2 out]
                  n214 = Wait (ms)(milliseconds to wait=u32 5000) -> ()  [unwired: 1 out]
                  n215 = Open/Create/Replace File(file path (use dialog)=w580, operation (0:open)=T4."open") -> (refnum out=w585:refnum<file>, error out=w584:errorcluster)  [unwired: 2 in, 3 out]
                  n216 = Set File Position(refnum=w585, from (0:start)=enum16{"start", "end", "current"}."end", error in=w584) -> (refnum out=w587:refnum<file>, error out=w588:errorcluster)  [unwired: 1 in]
                  n217 = call "RLC_read.vi"("Path"=path "H:/CDH/CDH_control/python_CDH", "String"="cmd /c rlc_read_ZCL.py") -> ("MEASURE A"=w571:dbl, "MEASURE V [V]"=w573:dbl, "concatenated string"=w594:string, "MEASURE B"=w574:dbl, "MEASURE I [A]"=w572:dbl)  [unwired: 1 out]
                  "MEASURE A 13" <- w571
                  "MEASURE B 13" <- w574
                  "MEASURE V [V]  13" <- w573
                  "MEASURE I [A]   13" <- w572
                  n218 = Number To Engineering String(2:w591, 4:w572) -> (0:w576:string)  [unwired: 2 in]
                  n219 = local write "RLC300 - digimess"(w594) -> ()
                  n220 = Number To Engineering String(2:w591, 4:w573) -> (0:w577:string)  [unwired: 2 in]
                  n221 = Number To Engineering String(2:w591, 4:w571) -> (0:w579:string)  [unwired: 2 in]
                  n222 = Number To Engineering String(2:w591, 4:w574) -> (0:w578:string)  [unwired: 2 in]
                  n223 = Concatenate Strings(w579, w575, w578, w575, w577, w575, w576, w575) -> (w581:string)
                  n224 = Write to Text File(file (use dialog)=w587, text=w581, error in=w588) -> (refnum out=w583:refnum<file>, error out=w582:errorcluster)  [unwired: 1 in, 1 out]
                  n225 = Close File(refnum=w583, error in=w582) -> (error out=w590:errorcluster)  [unwired: 1 out]
                  n226 = call <vilib>:"Simple Error Handler.vi"("error in (no error)"=w590) -> ()  [unwired: 1 in, 8 out]
                  "Z-1K-L" <- w592
                }
                frame #14 {
                  w601 = "\t"
                  w617 = i16 4 ("width (-)")
                  n227 = property on="path RLC" class="Path"() -> ("Value"=w606:path)  [unwired: 2 in, 2 out]
                  n228 = Wait (ms)(milliseconds to wait=u32 5000) -> ()  [unwired: 1 out]
                  n229 = Open/Create/Replace File(file path (use dialog)=w606, operation (0:open)=T4."open") -> (refnum out=w611:refnum<file>, error out=w610:errorcluster)  [unwired: 2 in, 3 out]
                  n230 = Set File Position(refnum=w611, from (0:start)=enum16{"start", "end", "current"}."end", error in=w610) -> (refnum out=w613:refnum<file>, error out=w614:errorcluster)  [unwired: 1 in]
                  n231 = call "RLC_read.vi"("Path"=path "H:/CDH/CDH_control/python_CDH", "String"="cmd /c rlc_read_ZCN.py") -> ("MEASURE A"=w597:dbl, "MEASURE V [V]"=w599:dbl, "concatenated string"=w620:string, "MEASURE B"=w600:dbl, "MEASURE I [A]"=w598:dbl)  [unwired: 1 out]
                  "MEASURE A 14" <- w597
                  "MEASURE B 14" <- w600
                  "MEASURE V [V]  14" <- w599
                  "MEASURE I [A]   14" <- w598
                  n232 = Number To Engineering String(2:w617, 4:w598) -> (0:w602:string)  [unwired: 2 in]
                  n233 = local write "RLC300 - digimess"(w620) -> ()
                  n234 = Number To Engineering String(2:w617, 4:w599) -> (0:w603:string)  [unwired: 2 in]
                  n235 = Number To Engineering String(2:w617, 4:w597) -> (0:w605:string)  [unwired: 2 in]
                  n236 = Number To Engineering String(2:w617, 4:w600) -> (0:w604:string)  [unwired: 2 in]
                  n237 = Concatenate Strings(w605, w601, w604, w601, w603, w601, w602, w601) -> (w607:string)
                  n238 = Write to Text File(file (use dialog)=w613, text=w607, error in=w614) -> (refnum out=w609:refnum<file>, error out=w608:errorcluster)  [unwired: 1 in, 1 out]
                  n239 = Close File(refnum=w609, error in=w608) -> (error out=w616:errorcluster)  [unwired: 1 out]
                  n240 = call <vilib>:"Simple Error Handler.vi"("error in (no error)"=w616) -> ()  [unwired: 1 in, 8 out]
                  "Z-1K-N" <- w618
                }
                frame #15 {
                  w627 = "\t"
                  w643 = i16 4 ("width (-)")
                  n241 = property on="path RLC" class="Path"() -> ("Value"=w632:path)  [unwired: 2 in, 2 out]
                  n242 = Wait (ms)(milliseconds to wait=u32 5000) -> ()  [unwired: 1 out]
                  n243 = Open/Create/Replace File(file path (use dialog)=w632, operation (0:open)=T4."open") -> (refnum out=w637:refnum<file>, error out=w636:errorcluster)  [unwired: 2 in, 3 out]
                  n244 = Set File Position(refnum=w637, from (0:start)=enum16{"start", "end", "current"}."end", error in=w636) -> (refnum out=w639:refnum<file>, error out=w640:errorcluster)  [unwired: 1 in]
                  n245 = call "RLC_read.vi"("Path"=path "H:/CDH/CDH_control/python_CDH", "String"="cmd /c rlc_read_ZDL.py") -> ("MEASURE A"=w623:dbl, "MEASURE V [V]"=w625:dbl, "concatenated string"=w646:string, "MEASURE B"=w626:dbl, "MEASURE I [A]"=w624:dbl)  [unwired: 1 out]
                  "MEASURE A 15" <- w623
                  "MEASURE B 15" <- w626
                  "MEASURE V [V]  15" <- w625
                  "MEASURE I [A]   15" <- w624
                  n246 = Number To Engineering String(2:w643, 4:w624) -> (0:w628:string)  [unwired: 2 in]
                  n247 = local write "RLC300 - digimess"(w646) -> ()
                  n248 = Number To Engineering String(2:w643, 4:w625) -> (0:w629:string)  [unwired: 2 in]
                  n249 = Number To Engineering String(2:w643, 4:w623) -> (0:w631:string)  [unwired: 2 in]
                  n250 = Number To Engineering String(2:w643, 4:w626) -> (0:w630:string)  [unwired: 2 in]
                  n251 = Concatenate Strings(w631, w627, w630, w627, w629, w627, w628, w627) -> (w633:string)
                  n252 = Write to Text File(file (use dialog)=w639, text=w633, error in=w640) -> (refnum out=w635:refnum<file>, error out=w634:errorcluster)  [unwired: 1 in, 1 out]
                  n253 = Close File(refnum=w635, error in=w634) -> (error out=w642:errorcluster)  [unwired: 1 out]
                  n254 = call <vilib>:"Simple Error Handler.vi"("error in (no error)"=w642) -> ()  [unwired: 1 in, 8 out]
                  "Z-10K-L" <- w644
                }
                frame #16 {
                  w654 = "\t"
                  w670 = i16 4 ("width (-)")
                  n255 = property on="path RLC" class="Path"() -> ("Value"=w659:path)  [unwired: 2 in, 2 out]
                  n256 = Wait (ms)(milliseconds to wait=u32 5000) -> ()  [unwired: 1 out]
                  n257 = Open/Create/Replace File(file path (use dialog)=w659, operation (0:open)=T4."open") -> (refnum out=w664:refnum<file>, error out=w663:errorcluster)  [unwired: 2 in, 3 out]
                  n258 = Set File Position(refnum=w664, from (0:start)=enum16{"start", "end", "current"}."end", error in=w663) -> (refnum out=w666:refnum<file>, error out=w667:errorcluster)  [unwired: 1 in]
                  n259 = call "RLC_read.vi"("Path"=path "H:/CDH/CDH_control/python_CDH", "String"="cmd /c rlc_read_ZDN.py") -> ("MEASURE A"=w649:dbl, "MEASURE V [V]"=w652:dbl, "concatenated string"=w673:string, "MEASURE B"=w653:dbl, "MEASURE I [A]"=w651:dbl)  [unwired: 1 out]
                  "MEASURE A 16" <- w649
                  "MEASURE B 16" <- w653
                  "MEASURE V [V]  16" <- w652
                  "MEASURE I [A]   16" <- w651
                  n260 = Number To Engineering String(2:w670, 4:w651) -> (0:w655:string)  [unwired: 2 in]
                  n261 = local write "RLC300 - digimess"(w673) -> ()
                  n262 = Number To Engineering String(2:w670, 4:w652) -> (0:w656:string)  [unwired: 2 in]
                  n263 = Number To Engineering String(2:w670, 4:w649) -> (0:w658:string)  [unwired: 2 in]
                  n264 = Number To Engineering String(2:w670, 4:w653) -> (0:w657:string)  [unwired: 2 in]
                  n265 = Concatenate Strings(w658, w654, w657, w654, w656, w654, w655, w654, "\r\n") -> (w660:string)
                  n266 = Write to Text File(file (use dialog)=w666, text=w660, error in=w667) -> (refnum out=w662:refnum<file>, error out=w661:errorcluster)  [unwired: 1 in, 1 out]
                  n267 = Close File(refnum=w662, error in=w661) -> (error out=w669:errorcluster)  [unwired: 1 out]
                  n268 = call <vilib>:"Simple Error Handler.vi"("error in (no error)"=w669) -> ()  [unwired: 1 in, 8 out]
                  "Z-10K-N" <- w671
                }
                frame #17 {
                  n269 = local write "Z-50-L"(w677) -> ()
                  n270 = local write "Z-100-L"(w677) -> ()
                  n271 = local write "Z-100-N"(w677) -> ()
                  n272 = local write "Z-10K-L"(w677) -> ()
                  n273 = local write "Z-10K-N"(w677) -> ()
                  n274 = local write "Z-1K-L"(w677) -> ()
                  n275 = local write "Z-1K-N"(w677) -> ()
                  n276 = local write "C-50-N"(w677) -> ()
                  n277 = local write "C-50-L"(w677) -> ()
                  n278 = local write "Z-50-N"(w677) -> ()
                  n279 = local write "C-1K-N"(w677) -> ()
                  n280 = local write "C-1K-L"(w677) -> ()
                  n281 = local write "C-10K-N"(w677) -> ()
                  n282 = local write "C-10K-L"(w677) -> ()
                  n283 = local write "C-100-N"(w677) -> ()
                  n284 = local write "C-100-L"(w677) -> ()
                }
              }
            }
            n285 = call <vilib>:"Mean.vi"("X"=w195) -> ("mean"=→"mean 14":dbl)  [unwired: 1 out]
            n286 = call <vilib>:"Mean.vi"("X"=w194) -> ("mean"=→"mean 15":dbl)  [unwired: 1 out]
            n287 = call <vilib>:"Mean.vi"("X"=w208) -> ("mean"=→"mean":dbl)  [unwired: 1 out]
            n288 = call <vilib>:"Mean.vi"("X"=w207) -> ("mean"=→"mean 2":dbl)  [unwired: 1 out]
            n289 = call <vilib>:"Mean.vi"("X"=w206) -> ("mean"=→"mean 3":dbl)  [unwired: 1 out]
            n290 = call <vilib>:"Mean.vi"("X"=w205) -> ("mean"=→"mean 4":dbl)  [unwired: 1 out]
            n291 = call <vilib>:"Mean.vi"("X"=w204) -> ("mean"=→"mean 5":dbl)  [unwired: 1 out]
            n292 = call <vilib>:"Mean.vi"("X"=w203) -> ("mean"=→"mean 6":dbl)  [unwired: 1 out]
            n293 = call <vilib>:"Mean.vi"("X"=w202) -> ("mean"=→"mean 7":dbl)  [unwired: 1 out]
            n294 = call <vilib>:"Mean.vi"("X"=w201) -> ("mean"=→"mean 8":dbl)  [unwired: 1 out]
            n295 = call <vilib>:"Mean.vi"("X"=w200) -> ("mean"=→"mean 9":dbl)  [unwired: 1 out]
            n296 = call <vilib>:"Mean.vi"("X"=w199) -> ("mean"=→"mean 10":dbl)  [unwired: 1 out]
            n297 = call <vilib>:"Mean.vi"("X"=w198) -> ("mean"=→"mean 11":dbl)  [unwired: 1 out]
            n298 = call <vilib>:"Mean.vi"("X"=w197) -> ("mean"=→"mean 12":dbl)  [unwired: 1 out]
            n299 = call <vilib>:"Mean.vi"("X"=w196) -> ("mean"=→"mean 13":dbl)  [unwired: 1 out]
            n300 = call <vilib>:"Mean.vi"("X"=w193) -> ("mean"=→"mean 16":dbl)  [unwired: 1 out]
          }
        }
        n301 = case shown="True" "Ligar RLC" {
          frame False {
          }
          frame True {
            n302 = call "RLC_open.vi"() -> ("String 2"=w679:string)  [unwired: 10 in, 1 out]
            n303 = local write "RLC300 - digimess"(w679) -> ()
          }
        }
        n304 = case shown="True" "Ligar RLC" {
          frame False {
          }
          frame True {
            w125 = "\t"
            w146 = "\t"
            w129 = "\r"
            w167 = "\r"
            w156 = "\t"
            n305 = Concatenate Strings("SET" ("Nota 4"), w125, "DATE" ("Nota 4"), w125, "TIME" ("Nota 4"), w125, w146, "P (BAR)" ("Nota 4"), w146, "T (ºC)" ("Nota 4"), w146, "C-50-L" ("Nota 4"), w146, "C-50-N" ("Nota 4"), w146, "C-100-L" ("Nota 4"), w146, "C-100-N" ("Nota 4"), w146, "C-1K-L" ("Nota 4"), w146, "C-1K-N" ("Nota 4"), w146, "C-10K-L" ("Nota 4"), w146, "C-10K-N" ("Nota 4"), w146, "Z-50-L" ("Nota 4"), w146, "Z-50-N" ("Nota 4"), w146, "Z-100-L" ("Nota 4"), w146, "Z-100-N" ("Nota 4"), w146, "Z-1K-L" ("Nota 4"), w146, "Z-1K-N" ("Nota 4"), w146, "Z-10K-L" ("Nota 4"), w146, "Z-10K-N" ("Nota 4")) -> (w130:string)
            n306 = Get Date/Time String(date format (0)=enum16{"short", "long", "abbreviated"}."short", want seconds? (F)=TRUE) -> (date string=w174:string, time string=w173:string)  [unwired: 1 in]
            n307 = property on="Sample name" class="Str"() -> ("Value"=w152:string)  [unwired: 2 in, 2 out]
            n308 = Concatenate Strings(w174, w156, w173) -> (w169:string)
            n309 = property on="File name" class="Str"() -> ("Value"=w151:string)  [unwired: 2 in, 2 out]
            n310 = Concatenate Strings(w151, " RLC_CDH" ("string")) -> (w149:string)
            n311 = Concatenate Strings("Sievert RLC - CDH:" ("string"), w156, w152, "\r\n") -> (w154:string)
            n312 = Concatenate Strings("Data Table" ("string"), w129, "==========" ("string"), w129, w130, w129) -> (w168:string)
            n313 = File Dialog(6:".txt" ("pattern label"), 9:w149) -> (0:w165:errorcluster, 3:w166:path)  [unwired: 2 in, 5 out]
            n314 = Open/Create/Replace File(file path (use dialog)=w166, error in=w165, operation (0:open)=T4."replace or create with confirmation", access (0:read/write)=enum16{"read/write", "read-only", "write-only"}."read/write") -> (refnum out=w162:refnum<file>, error out=w161:errorcluster)  [unwired: 3 out]
            n315 = Concatenate Strings(w169, w167, w167, w154, w167, w167, "Nota 01: MEDIDAS COM RLC 300 - MULTILEITURA" ("Nota 4"), w167, w167, w168) -> (w172:string)
            n316 = Write to Text File(file (use dialog)=w162, text=w172, error in=w161) -> (refnum out=w160:refnum<file>, error out=w158:errorcluster)  [unwired: 1 in, 1 out]
            n317 = Close File(refnum=w160, error in=w158) -> (path=w153:path)  [unwired: 1 out]
            n318 = local write "path RLC"(w153) -> ()
          }
        }
        n319 = case shown="True" "Close RLC 2" {
          frame False {
          }
          frame True {
            n320 = call "RLC_close.vi"() -> ("String"=w678:string)  [unwired: 11 in]
            n321 = local write "RLC300 - digimess"(w678) -> ()
          }
        }
        n322 = Or(x=w57, y="Refresh Button") -> (x .or. y?=w58:bool)
        n323 = case shown="True" w58 {
          frame False {
          }
          frame True {
            n324 = stacked-sequence {
              frame #0 {
                n325 = property on="Waveform Chart P 2" class="WFChart (strict)"("History Data"=dbl[][] []) -> ()  [unwired: 2 in, 2 out]
                n326 = property on="Waveform Chart P 3" class="WFChart (strict)"("History Data"=dbl[][] []) -> ()  [unwired: 2 in, 2 out]
              }
              frame #1 {
                n327 = property on="path RLC" class="Path"() -> ("Value"=w80:path)  [unwired: 2 in, 2 out]
                n328 = Open/Create/Replace File(file path (use dialog)=w80, operation (0:open)=T4."open", access (0:read/write)=enum16{"read/write", "read-only", "write-only"}."read-only") -> (refnum out=w79:refnum<file>, error out=w78:errorcluster)  [unwired: 3 in, 1 out]
                n329 = Read from Text File(file (use dialog)=w79, error in=w78) -> (refnum out=w85:refnum<file>, text=w81:string, error out=w84:errorcluster)  [unwired: 2 in, 1 out]
                n330 = Close File(refnum=w85, error in=w84) -> ()  [unwired: 2 out]
                n331 = Search/Split String(string=w81, search string/char (-)="SET\tDATE\tTIME\t\tP (BAR)\tT (ºC)\tC-50-L\tC-50-N\tC-100-L\tC-100-N\tC-1K-L\tC-1K-N\tC-10K-L\tC-10K-N\tZ-50-L\tZ-50-N\tZ-100-L\tZ-100-N\tZ-1K-L\tZ-1K-N\tZ-10K-L\tZ-10K-N") -> (match + rest of string=w86:string)  [unwired: 1 in, 2 out]
                n332 = String Subset(string=w86, offset (0)=150) -> (substring=w99:string)  [unwired: 1 in]
                n333 = Spreadsheet String To Array(delimiter (Tab)="", format string="%t", spreadsheet string=w99) -> (array=w96:dbl[][])  [unwired: 1 in]
                n334 = Spreadsheet String To Array(format string="%#g", spreadsheet string=w99) -> (array=w92:dbl[][])  [unwired: 2 in]
                n335 = Transpose Matrix(1:w96) -> (0:w97:dbl[][])
                n336 = Transpose Matrix(1:w92) -> (0:w112:dbl[][])
                n337 = Index Array(array=w97, index (row)=0 ("index (row) 2")) -> (element=→"t":dbl[])  [unwired: 1 in]
                n338 = Index Array(array=w112, index (row)=5 ("index (row) 4")) -> (element=w113:dbl[])  [unwired: 1 in]
                n339 = Index Array(array=w112, index (row)=9 ("index (row) 5")) -> (element=w114:dbl[])  [unwired: 1 in]
                n340 = Index Array(array=w112, index (row)=37 ("index (row) 4")) -> (element=w73:dbl[])  [unwired: 1 in]
                n341 = Index Array(array=w112, index (row)=41 ("index (row) 5")) -> (element=w72:dbl[])  [unwired: 1 in]
                n342 = Index Array(array=w112, index (row)=45 ("index (row) 2")) -> (element=w71:dbl[])  [unwired: 1 in]
                n343 = Index Array(array=w112, index (row)=49 ("index (row) 3")) -> (element=w70:dbl[])  [unwired: 1 in]
                n344 = Index Array(array=w112, index (row)=53 ("index (row) 4")) -> (element=w69:dbl[])  [unwired: 1 in]
                n345 = Index Array(array=w112, index (row)=57 ("index (row) 5")) -> (element=w68:dbl[])  [unwired: 1 in]
                n346 = Index Array(array=w112, index (row)=61 ("index (row) 2")) -> (element=w67:dbl[])  [unwired: 1 in]
                n347 = Index Array(array=w112, index (row)=65 ("index (row) 3")) -> (element=w66:dbl[])  [unwired: 1 in]
                n348 = Index Array(array=w112, index (row)=13 ("index (row) 2")) -> (element=w115:dbl[])  [unwired: 1 in]
                n349 = Index Array(array=w112, index (row)=17 ("index (row) 3")) -> (element=w116:dbl[])  [unwired: 1 in]
                n350 = Index Array(array=w112, index (row)=21 ("index (row) 4")) -> (element=w117:dbl[])  [unwired: 1 in]
                n351 = Index Array(array=w112, index (row)=25 ("index (row) 5")) -> (element=w118:dbl[])  [unwired: 1 in]
                n352 = Index Array(array=w112, index (row)=29 ("index (row) 2")) -> (element=w119:dbl[])  [unwired: 1 in]
                n353 = Index Array(array=w112, index (row)=33 ("index (row) 3")) -> (element=w120:dbl[])  [unwired: 1 in]
                n354 = Build Array(w73, w72, w71, w70, w69, w68, w67, w66) -> (w75:dbl[][])
                n355 = Build Array(w113, w114, w115, w116, w117, w118, w119, w120) -> (w121:dbl[][])
                n356 = Transpose Matrix(1:w75) -> (0:→"Waveform Chart P 3" →"appended array 2":dbl[][])
                n357 = Transpose Matrix(1:w121) -> (0:→"Waveform Chart P 2" →"appended array":dbl[][])
              }
            }
          }
        }
      }
    }
    n358 = case shown="False" "Save Data" {
      frame False {
      }
      frame True {
        n359 = property on="path" class="Path"() -> ("Value"=w681:path)  [unwired: 2 in, 2 out]
        n360 = Open/Create/Replace File(file path (use dialog)=w681, operation (0:open)=T4."open") -> (refnum out=w686:refnum<file>, error out=w685:errorcluster)  [unwired: 2 in, 3 out]
        n361 = Set File Position(refnum=w686, from (0:start)=enum16{"start", "end", "current"}."end", error in=w685) -> (refnum out=w688:refnum<file>, error out=w689:errorcluster)  [unwired: 1 in]
        n362 = Write to Text File(file (use dialog)=w688, text="dados", error in=w689) -> (refnum out=w684:refnum<file>, error out=w683:errorcluster)  [unwired: 1 in, 1 out]
        n363 = Close File(refnum=w684, error in=w683) -> (error out=w691:errorcluster)  [unwired: 1 out]
        n364 = call <vilib>:"Simple Error Handler.vi"("error in (no error)"=w691) -> ()  [unwired: 1 in, 8 out]
      }
    }
    n365 = case shown="False" "New" {
      frame False {
      }
      frame True {
        w708 = "\t"
        w712 = "\r"
        w710 = "\t"
        w718 = "\r"
        w715 = "\r"
        w695 = "\t"
        n366 = Concatenate Strings("Nota 01:" ("Nota 4"), w710, "Nota 01", w712, "Nota 02:" ("Nota 4"), w710, "Nota 2", w712, "Nota 03:" ("Nota 4"), w710, "Nota 3") -> (w709:string)
        n367 = File Dialog(6:".txt" ("pattern label"), 9:"File name") -> (0:w705:errorcluster, 3:w706:path)  [unwired: 2 in, 5 out]
        n368 = Get Date/Time String(date format (0)=enum16{"short", "long", "abbreviated"}."short", want seconds? (F)=TRUE) -> (date string=w728:string, time string=w727:string)  [unwired: 1 in]
        n369 = Concatenate Strings(w728, w695, w727) -> (w717:string)
        n370 = Concatenate Strings("Data Table" ("string"), w718, "==========" ("string"), w718, "data   time" ("string"), w708, "         " ("string"), w708, "P (bar)" ("string"), w708, "T (ºC)    " ("string"), w708, "  " ("string"), "\r\n") -> (w716:string)
        n371 = Concatenate Strings("Arduino UNO Sievert 01:" ("string"), w695, "Sample name", "\r\n") -> (w693:string)
        n372 = Open/Create/Replace File(file path (use dialog)=w706, error in=w705, operation (0:open)=T4."replace or create with confirmation", access (0:read/write)=enum16{"read/write", "read-only", "write-only"}."read/write") -> (refnum out=w702:refnum<file>, error out=w701:errorcluster)  [unwired: 3 out]
        n373 = Concatenate Strings(w717, w715, w715, w693, w715, w715, w709, w715, w715, w716) -> (w726:string)
        n374 = Write to Text File(file (use dialog)=w702, text=w726, error in=w701) -> (refnum out=w700:refnum<file>, error out=w698:errorcluster)  [unwired: 1 in, 1 out]
        n375 = Close File(refnum=w700, error in=w698) -> (path=w692:path)  [unwired: 1 out]
        n376 = local write "path"(w692) -> ()
      }
    }
    n377 = Unbundle By Name(w55) -> ("status"=w53:bool)
    n378 = Get Date/Time String(date format (0)=enum16{"short", "long", "abbreviated"}."short", want seconds? (F)=TRUE) -> (date string=w26:string, time string=w25:string)  [unwired: 1 in]
    n379 = Multiply(x="Time (sec)", y=1000.0) -> (x*y=w32:dbl)
    n380 = case shown="False" "New Button" {
      frame False {
      }
      frame True {
        w680 = dynamicdata[] [] ("History Data")
        n381 = property on="Waveform Chart T" class="WFChart (strict)"("History Data"=w680) -> ()  [unwired: 2 in, 2 out]
        n382 = property on="Waveform Chart P" class="WFChart (strict)"("History Data"=w680) -> ()  [unwired: 2 in, 2 out]
      }
    }
    n383 = Concatenate Strings(w26, w17, w25, w17) -> (w24:string)
    n384 = Index Array(array=w49, index="Analog Pin A") -> (element=w45:dbl)
    "Voltage A" <- w45
    n385 = Index Array(array=w49, index="Analog Pin B") -> (element=w41:dbl)
    "Voltage B" <- w41
    n386 = Index Array(array=w49, index="Analog Pin C") -> (element=w15:dbl)
    "Voltage C" <- w15
    n387 = Wait Until Next ms Multiple(millisecond multiple=w32) -> ()  [unwired: 1 out]
    n388 = Or(x=w53, y="Stop") -> (x .or. y?=w54:bool)
    n389 = Subtract "ddp(V)"(x=w45, y=w41) -> (x-y=w44:dbl)
    n390 = Multiply(x=w15, y="Ajute P") -> (x*y=w23:dbl)
    "Pressure (bar)" <- w23
    n391 = Merge Signals(w15) -> (→"Waveform Chart 2":dynamicdata)
    n392 = formula code="float a;\na=(ddp/5)+0.5;\nfloat b;\nb=0.5-(ddp/5);\nr=100*(a/b)-0.756;\nfloat AA;\nfloat BB;\nfloat CC;\nfloat DD;\nfloat EE;\nfloat FF;\nAA=-242.02;\nBB=2.22280;\nCC=0.0025859;\nDD=-0.000004826;\nEE=-0.0000000281830;\nFF=0.000000000152430;\nt=AA+BB*r+CC*(r**2)+DD*(r**3)+EE*(r**4)+FF*(r**5);"("ddp"=w44) -> ("r"=w43:dbl, "t"=w34:dbl)
    "Resistencia" <- w43
    "Temperatura" <- w34
    n393 = Number To Engineering String(2:w16, 4:w23) -> (0:w21:string)  [unwired: 2 in]
    n394 = Merge Signals(w23) -> (→"Waveform Chart P":dynamicdata)
    n395 = Merge Signals(w43, w34) -> (→"Waveform Chart":dynamicdata)
    n396 = Add(x=w34, y="Ajute T") -> (x+y=w22:dbl)
    "Temperature (ºC)" <- w22
    n397 = Number To Engineering String(2:w16, 4:w22) -> (0:w20:string)  [unwired: 2 in]
    n398 = Merge Signals(w22) -> (→"Waveform Chart T":dynamicdata)
    n399 = Concatenate Strings(w24, w21, w17, w20, "\r\n") -> (w18:string)
    n400 = local write "dados"(w18) -> ()
  }
  n401 = local write "Analog Pin A"(Analog_Pin."Anlog In 0" ("Analog Pin A")) -> ()
  n402 = local write "Analog Pin B"(Analog_Pin."Anlog In 1" ("Analog Pin B")) -> ()
  n403 = local write "Analog Pin C"(Analog_Pin."Anlog In 2" ("Analog Pin C")) -> ()
  n404 = local write "path"(path "H:/teste_arquivo.txt" ("path")) -> ()
  n405 = call <vilib>:"Close.vi"("Arduino Resource"=w12, "error in"=w11) -> ("error out"=w9:errorcluster)  [unwired: 13 in]
  n406 = call <vilib>:"Simple Error Handler.vi"("error in (no error)"=w9) -> ()  [unwired: 4 in, 5 out]
